vi "Interfaz grafica - corriente(1).vi"() -> ()   [LabVIEW 2016]
uses:
  Optotune Lens Driver 4 Labview package/Optotune Lens Driver 4 Labview package/Hello Optotune Lens (30.06.2015)/Calibration.ctl
  <vilib>/DAQmx/read.llb/DAQmx Read (Analog 1D Wfm NChan NSamp).vi
  <vilib>/Analysis/2dsp.llb/Decimate (single shot, DBL).vi
  <vilib>/Utility/file.llb/Read Delimited Spreadsheet (string).vi
  <vilib>/DAQmx/miscellaneous.llb/DAQmx Fill In Error Info.vi
  <vilib>/Waveform/WDTOps.llb/WDT Index Channel DBL.vi
  <vilib>/Analysis/2dsp.llb/Decimate (continuous, DBL).vi
  <vilib>/Instr/_visa.llb/VISA Configure Serial Port (Instr).vi
  <vilib>/Utility/file.llb/Write Delimited Spreadsheet (string).vi
  <vilib>/Waveform/WDTOps.llb/WDT Get Waveform Time Array DBL.vi
  <vilib>/Analysis/NI_AALPro.lvlib
panel:
  in  "Restablecer Iniciales":bool
  in  "Incremento":dbl=0.1 format="%#_13g"
  out "Potencia derecho":dbl
  out "error out 4":errorcluster
  out "error out 3":errorcluster
  out "error out 2":errorcluster
  in  "Tab Control 3":enum32{"WL", "Video"}(tab)
  out "Waveform length":dbl[][](graph)
  in  "Minimo escala Y":dbl format="%#_13g"
  in  "Maximo escala Y":dbl format="%#_13g"
  in  "Escala autom. Y":u8=1
  in  "Escala autom. X":u8=1
  in  "Maximo escala X":dbl
  in  "Minimo escala X":dbl
  out "Image Out":T1(plugin-control)
  in  "Frame Rate":u32=30
  in  "Modo de video":u16(ring)=21 items=["160x90 I420 30 fps", "160x90 MJPG 30 fps", "160x90 RGB24 30 fps", "160x120 I420 30 fps", "160x120 MJPG 30 fps", "160x120 RGB24 30 fps", "176x144 I420 30 fps", "176x144 MJPG 30 fps", "176x144 RGB24 30 fps", "320x180 I420 30 fps", "320x180 MJPG 30 fps", "320x180 RGB24 30 fps", "320x240  I420 30 fps", "320x240 MJPG 30 fps", "320x240 RGB24 30 fps", "352x288 I420 30 fps", "352x288 MJPG 30 fps", "352x288 RGB24 30 fps", "432x240 I420 30 fps", "432x240 MJPG 30 fps", "432x240 RGB24 30 fps", "640x360 I420 30 fps", "640x360 MJPG 30 fps", "640x360 RGB24 30 fps", "640x480 I420 30 fps", "640x480 MJPG 30 fps", "640x480 RGB24 30 fps", "800x448 I420 30 fps", "800x448 MJPG 30 fps", "800x448 RGB24 30 fps", "800x600 I420 30 fps", "800x600 MJPG 30 fps", "800x600 RGB24 30 fps", "864x480 I420 30 fps", "864x480 MJPG 30 fps", "864x480 RGB24 30 fps", "960x720 I420 30 fps", "960x720 MJPG 30 fps", "960x720 RGB24 30 fps", "1024x576 I420 30 fps", "1024x576 MJPG 30 fps", "1024x576 RGB24 30 fps", "1280x720 I420 30 fps", "1280x720 MJPG 30 fps", "1280x720 RGB24 30 fps", "1600x896 I420 30 fps", "1600x896 MJPG 30 fps", "1600x896 RGB24 30 fps", "1920x1080 I420 5 fps", "1920x1080 MJPG 30 fps", "1920x1080 RGB24 5 fps", "2304x1296 I420 2 fps", "2304x1296 RGB24 2 fps", "2304x1536 I420 2 fps", "2304x1536 RGB24 2 fps"]
  in  "Carpeta archivo":string="C:\\Users\\TGM1603\\Documents\\LabVIEW Data\\Experimentos electrodos\\VideosExperimentos"
  in  "Calidad":u32=1000
  out "VISA resource name out":string
  in  "Tab Control 2":T2(tab)
  in  "DAQmx Physical Channel":tag
  in  "Frecuencia muestreo":i32=20000
  in  "Rango voltaje":i16(ring)=5 items=["0.1"=0, "1"=1, "5"=5, "10"=10]
  in  "tamaño buffer":i32=1000
  in  "factor decimacion":i32=20
  in  "Ganancia":u16(ring) items=["0.2"=51455, "1"=33023, "10"=49407, "20"=41215, "30"=57599, "40"=37119, "60"=53503, "80"=45311, "120"=61695, "157"=35071, ""=0]
  in  "Potencia inicial lente derecho":dbl(slide) scale=-3.0..3.0
  in  "Potencia inicial lente izquierdo":dbl(slide) scale=-3.0..3.0
  in  "VISA resource name":string="COM11"
  in  "VISA resource name 2":string="COM10"
  out "DPT INICIALES D":dbl
  out "DPT INICIALES I":dbl
  out "Potencia izquierdo":dbl
  in  "error in (no error) 5":errorcluster
  in  "error in (no error) 4":errorcluster
  in  "error in (no error) 3":errorcluster
  in  "error in (no error) 2":errorcluster
  in  "Calibration 4":T3={"Max Current A"=293.0, "Max Current B"=293.0, "UCL A"=300.0, "UCL B"=300.0, "LCL A"=0.0, "LCL B"=0.0} {"Max Current A" format="%#_g mA"; "Max Current B" format="%#_g mA"; "UCL A" format="%#_g mA"; "LCL A" format="%#_g mA"; "UCL B" format="%#_g mA"; "LCL B" format="%#_g mA"}
  out "ID 2":u16
  out "VISA resource name out 2":string
  out "Calibration 3":T3 {"Max Current A" format="%#_g mA"; "Max Current B" format="%#_g mA"; "UCL A" format="%#_g mA"; "LCL A" format="%#_g mA"; "UCL B" format="%#_g mA"; "LCL B" format="%#_g mA"}
  out "OK 2":bool
  out "Data 2":string
  out "Command to Port 2":string
  in  "Cola tipo 2":dbl[](array[numeric])
  out "Distancia":u32
  in  "Tamaño ventana WL":i32=60
  in  "Limite inferior WL":dbl=25.0 format="%#_13g"
  in  "Limite superior WL":dbl=50.0
  out "number":u32
  in  "Calibration":T3={"Max Current A"=293.0, "Max Current B"=293.0, "UCL A"=300.0, "UCL B"=300.0, "LCL A"=0.0, "LCL B"=0.0} {"Max Current A" format="%#_g mA"; "Max Current B" format="%#_g mA"; "UCL A" format="%#_g mA"; "LCL A" format="%#_g mA"; "UCL B" format="%#_g mA"; "LCL B" format="%#_g mA"}
  out "ID":u16
  out "Calibration 2":T3 {"Max Current A" format="%#_g mA"; "Max Current B" format="%#_g mA"; "UCL A" format="%#_g mA"; "LCL A" format="%#_g mA"; "UCL B" format="%#_g mA"; "LCL B" format="%#_g mA"}
  out "OK":bool
  out "Data":string
  out "Command to Port":string
  in  "DPT dif.":dbl
  out "error out":errorcluster
  in  "error in (no error)":errorcluster
  in  "WL":dbl
  in  "Cola tipo":dbl[](array[numeric])
  out "T button?":bool
  in  "Elegir menu Exp":bool
  in  "Elegir menu":bool
  out "path":path
  in  "Iniciar experimento":bool
  in  "Parar adquisicion":bool
  out "Enfermedad visual":string
  out "Edad":string
  out "Nombre":string
  out "Cedula":string
  in  "Carpeta":path=path "C:/Users/TGM1603/Documents/LabVIEW Data/Experimentos electrodos"
  in  "?":bool
  in  "Menu Principal":u16(ring) items=["Visualizacion general ", "Llevar a cabo un experimento", "Ajustar potencia inicial lentes"]
  in  "Menu experimentos":u16(ring) items=["Experimento 1", "Experimento 2", "Experimento 3", "Experimento 4", "", "", "", ""]
  in  "Tab Control":enum32{"Señal EMG", "Potencia y distancia"}(tab)
  out "Senal EMG":waveform(dbl)[](graph)
  in  "Escala automatica Y":u8
  in  "Escala automatica X":u8=1
  in  "X Scale.Range:Increment":dbl
  in  "X Scale.Range:Minimum":dbl
  in  "X Scale.Range:Maximum":dbl
  in  "Y Scale.Range:Minimum":dbl=-5.0
  in  "Y Scale.Range:Maximum":dbl=5.0
  in  "Escala Y min":dbl
  in  "Escala Y max":dbl
  in  "Auto scale Y":u8=1
  in  "Escala X max":dbl
  in  "Escala X min":dbl
  out "Potencia optica y distancia":dbl[][](graph)
  in  "Auto scale X":u8=1
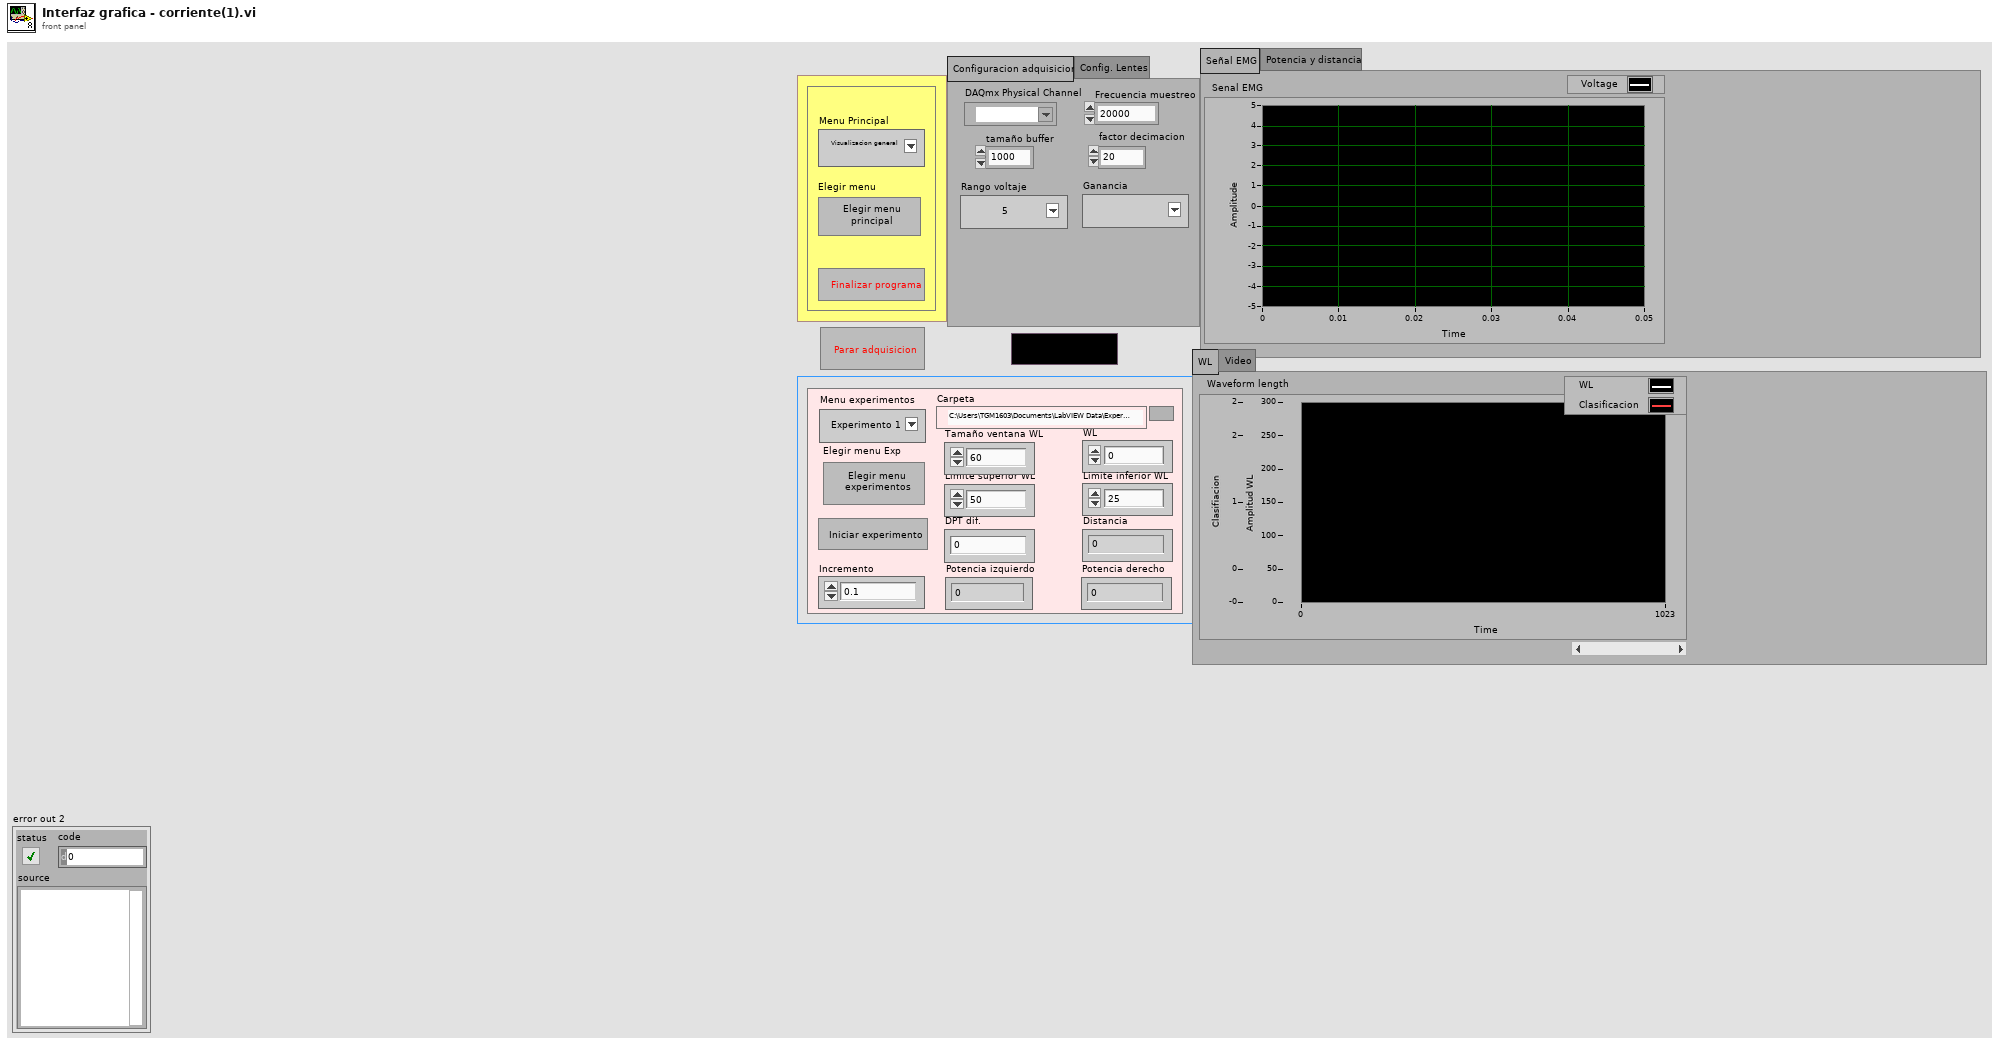
[diagram p1: front panel]
types:
  T1 = typedef "IMAQ Image.ctl" = refnum<image>
  T2 = enum32{"Configuracion adquisicion", "Config. Lentes"}
  T3 = typedef "Calibration.ctl" = cluster{"Max Current A":dbl, "Max Current B":dbl, "UCL A":dbl, "UCL B":dbl, "LCL A":dbl, "LCL B":dbl}
  T4 = enum16{"Left Button", "Center Button", "Right Button", "Window Close"}
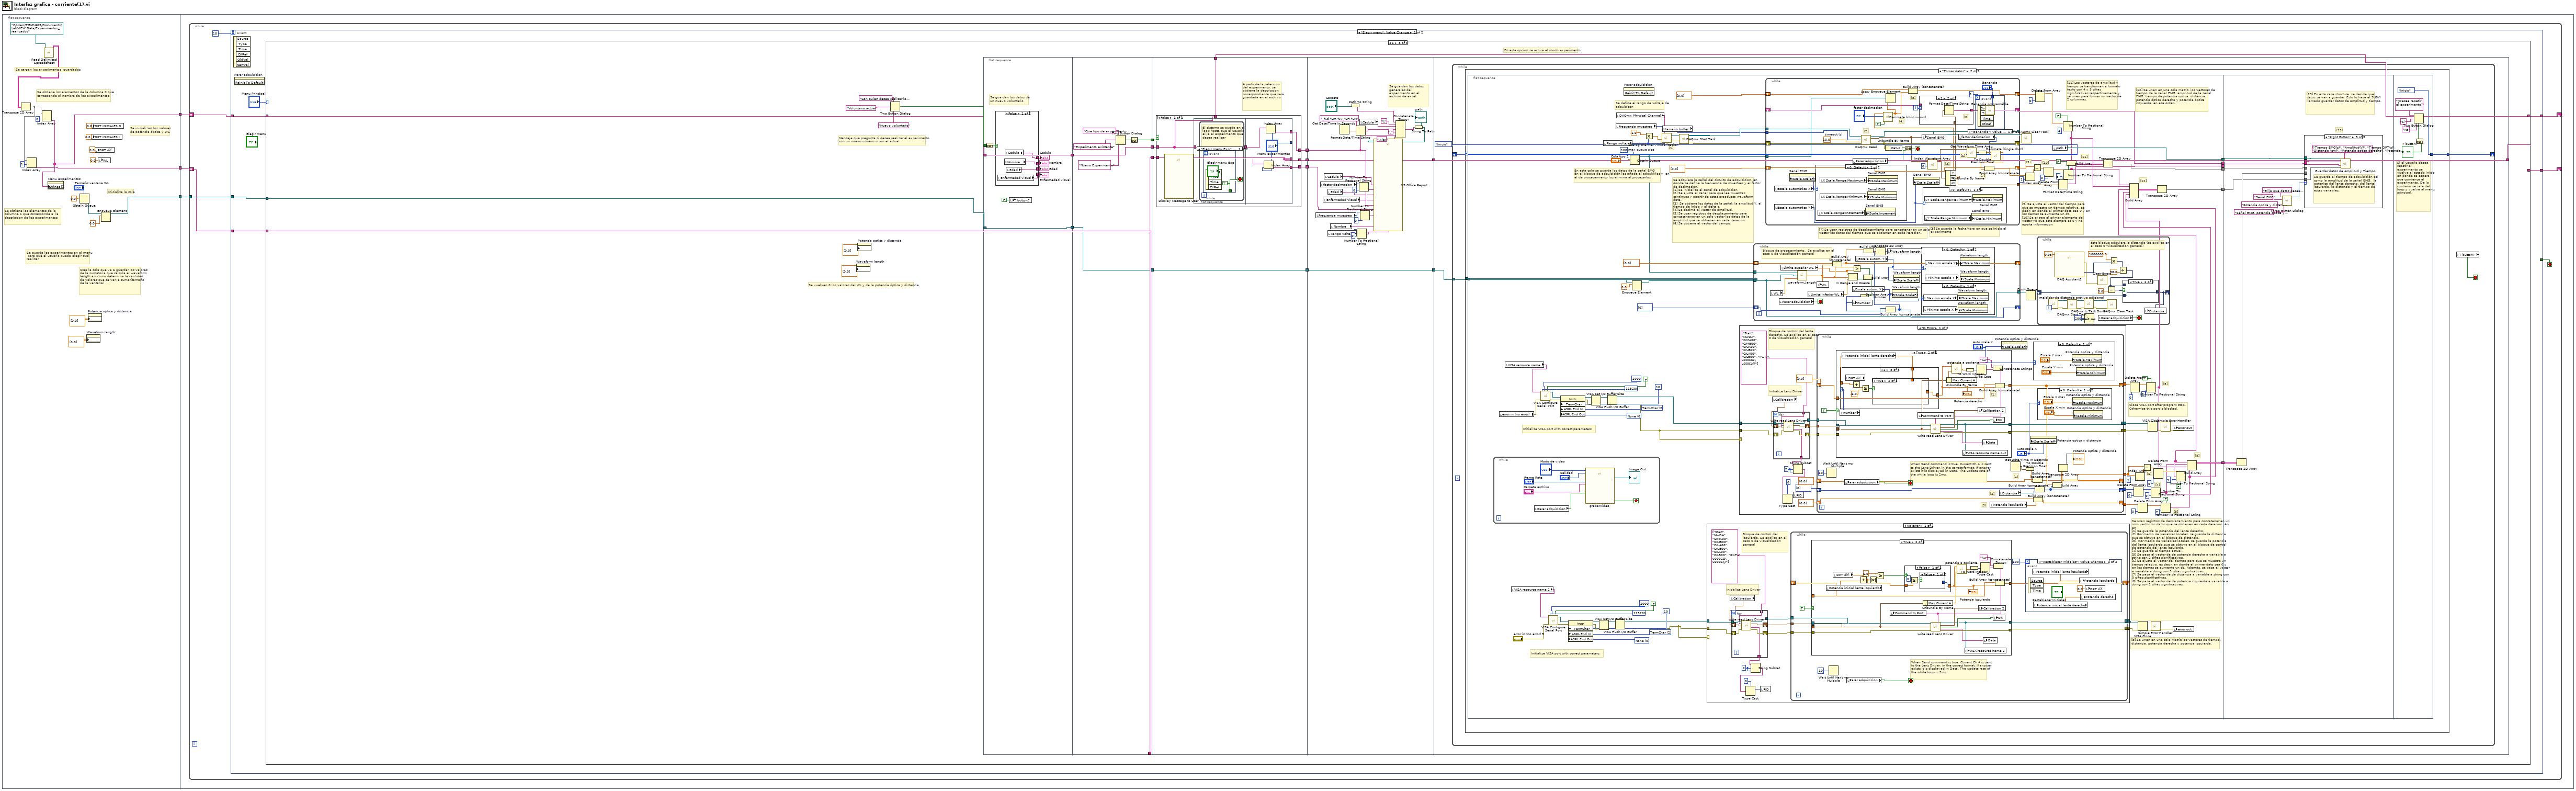
[diagram p0: block diagram]
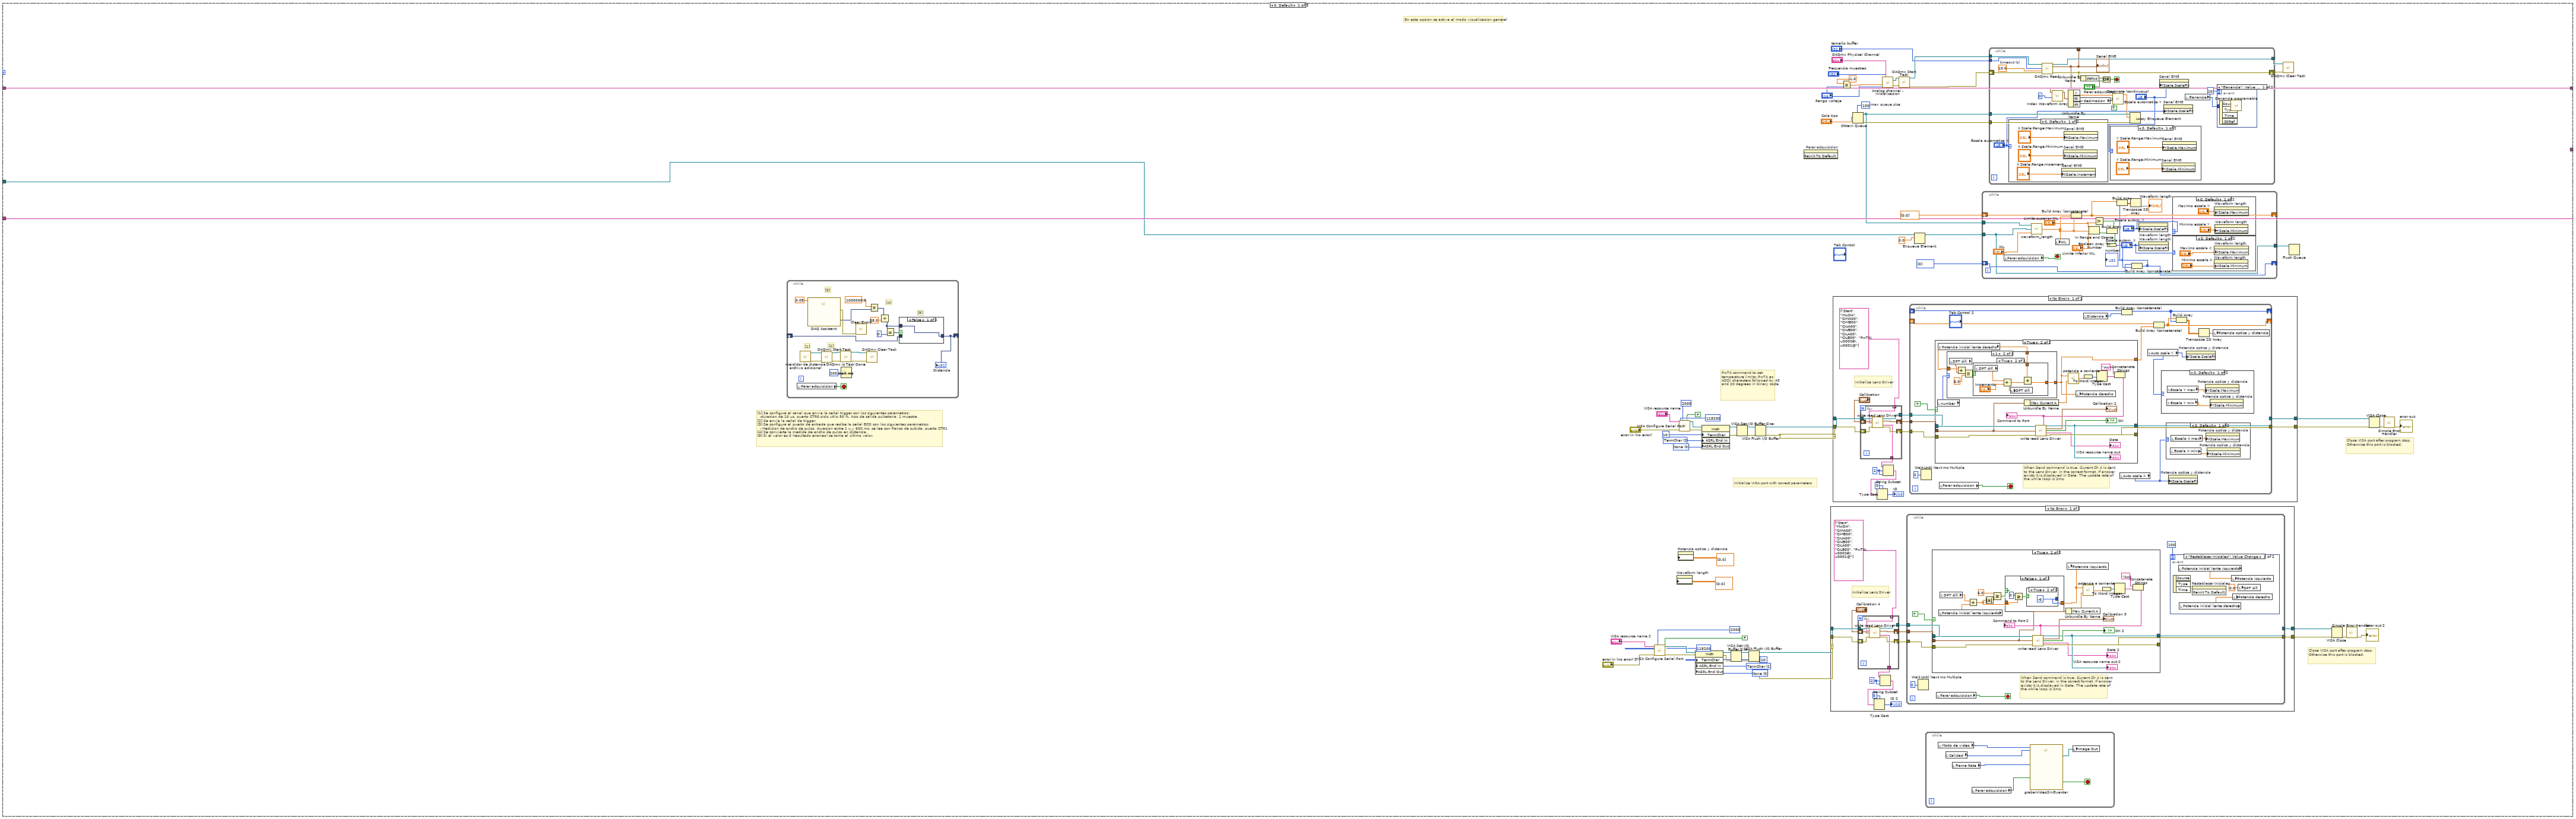
[diagram p2: hidden frame]
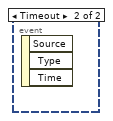
[diagram p3: hidden frame]
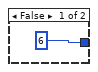
[diagram p5: hidden frame]
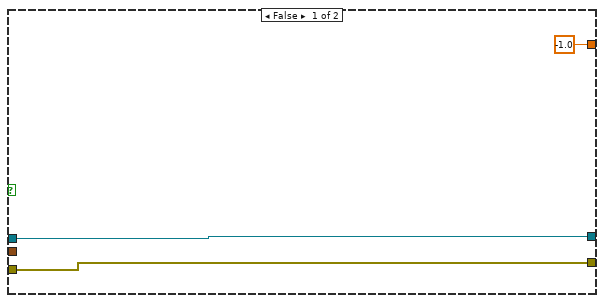
[diagram p11: hidden frame]
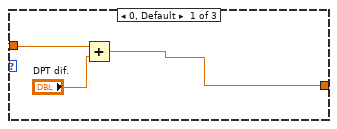
[diagram p12: hidden frame]
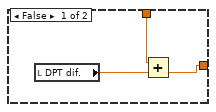
[diagram p13: hidden frame]
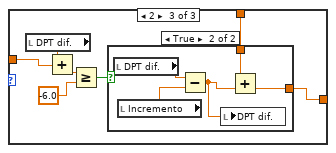
[diagram p14: hidden frame]
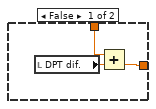
[diagram p15: hidden frame]
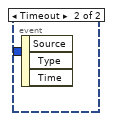
[diagram p19: hidden frame]
diagram:
  n1 = flat-sequence {
    tunnel: [w18] -> w3
    tunnel: [w15] -> w2
    tunnel: [w10] -> w1
    tunnel: w3 -> [w24]
    tunnel: w2 -> [w23]
    tunnel: w1 -> [w22]
    frame #0 {
      # "Se inicializan los valores\nde potencia óptica y WL"
      # "Inicializa la cola"
      # "Crea la cola que va a guardar los valores de la sumatoria que calcula el waveform length así como determina la cantidad de valores que se van a sumar(tamaño de la ventana)"
      # "Se obtiene los elementos de la columna 1 que corresponde a  la descripcion de los experimentos"
      # "Se obtiene los elementos de la columna 0 que corresponde al nombre de los experimentos"
      # "Se guarda los experimentos en el menu\n para que el usuario pueda elegir cual \nrealizar"
      # "Se cargan los experimentos  guardados"
      n2 = call-poly <vilib>:"Read Delimited Spreadsheet.vi"("file path (dialog if empty)"=path "C:/Users/TGM1603/Documents/LabVIEW Data/Experimentos_realizados") -> ("all rows"=w19:string[][])  [unwired: 9 in, 5 out]
      n3 = Transpose 2D Array(2D array=w19) -> (transposed array=w16:string[][])
      n4 = Index Array(array=w16, index (row)=1) -> (element=w15:string[])  [unwired: 1 in]
      n5 = Index Array(array=w16, index (row)=0) -> (element=w18:string[])  [unwired: 1 in]
      n6 = property on="Menu experimentos" class="Ring (strict)"("Strings []"=w18) -> ()  [unwired: 2 in, 2 out]
      n7 = Obtain Queue(max queue size (-1, unlimited)="Tamaño ventana WL", element data type=0.0) -> (queue out=w13:refnum<queue>)  [unwired: 3 in, 2 out]
      n8 = property on="Waveform length" class="WFChart (strict)"("History Data"=dbl[][] [[0.0]]) -> ()  [unwired: 2 in, 2 out]
      n9 = property on="Potencia optica y distancia" class="WFChart (strict)"("History Data"=dbl[][] [[0.0]]) -> ()  [unwired: 2 in, 2 out]
      n10 = local write "DPT INICIALES D"(0.0 ("DPT INIT.1")) -> ()
      n11 = local write "DPT INICIALES I"(0.0 ("DPT INIT.2")) -> ()
      n12 = local write "DPT dif."(0.0 ("WL")) -> ()
      n13 = local write "WL"(0.0 ("WL")) -> ()
      n14 = Enqueue Element(queue=w13, element=0.0) -> (queue out=w10:refnum<queue>)  [unwired: 2 in, 2 out]
    }
    frame #1 {
      n15 = while {
        shift-right: [w30] -> _
        shift-left: w24 -> [w31]
        shift-right: [w28] -> _
        shift-left: w23 -> [w29]
        tunnel: w22 -> [w27]
        stop <- w26 stop-if-true
        n16 = event shown="[0] \"Elegir menu\": Value Change" {
          selector: _ -> [_ _]
          dyn-events: _ -> [_ _]
          timeout: 10 -> [_ _]
          tunnel: w31 -> [w37 _]
          tunnel: [w36 _] -> w30
          tunnel: w29 -> [w35 _]
          tunnel: [w34 _] -> w28
          tunnel: w27 -> [w32 _]
          tunnel: [_ "?"] -> w26
          event "Elegir menu": Value Change {
            n17 = event-data() -> ()  [unwired: 1 in, 6 out]
            n18 = invoke on="Parar adquisicion" class="Bool (strict)" method="Reinit To Default"() -> ()  [unwired: 3 in, 3 out]
            n19 = case shown="1" "Menu Principal" {
              tunnel: w37 -> [w103 w388 w508]
              tunnel: [w103 w388 w507] -> w36
              tunnel: w35 -> [w102 w387 w505]
              tunnel: [w102 w387 w504] -> w34
              tunnel: w32 -> [w85 _ w495]
              frame 0, Default {
                w53 = u16 0 items=["None", "Last Bit", "TermChar", "Break"] ("Serial Settings:End Mode for Writes")
                w52 = u16 2 items=["None", "Last Bit", "TermChar"] ("Serial Settings:End Mode for Reads")
                w75 = u16 0 items=["None", "Last Bit", "TermChar", "Break"] ("Serial Settings:End Mode for Writes")
                w76 = u16 2 items=["None", "Last Bit", "TermChar"] ("Serial Settings:End Mode for Reads")
                w89 = 100  # max queue size
                # "En esta opcion se activa el modo visualizacion general"
                # "Close VISA port after program stop. Otherwise this port is blocked."
                # "[1] Se configura el canal que envía la señal trigger con los siguientes parametros:\n  -duracion de 10 us, puerto CTR0,ciclo utilo 50 %, tipo de salida pulsatoria, 1 muestra \n[2] Se envía la señal de trigger.\n[3] Se configura el puerto de entrada que recibe la señal ECO con los siguientes parámetros:\n  - Medicion de ancho de pulso, duracion entre 1 u y 600 ms, se lee con flanco de subida, puerto CTR1\n[4] Se convierte la medida de ancho de pulso en distancia.\n[5] Si el valor es 0 (resultado erroneo) se toma el último valor."
                # "PwTA command to set temperature limits: PwTA as ASCII characters followed by 45 and 20 degrees in binary code."
                # "Close VISA port after program stop. Otherwise this port is blocked."
                # "Initialize VISA port with correct parameters"
                n20 = while {
                  shift-right: [w177] -> _
                  shift-left: _ -> [w176]
                  stop <- w181 stop-if-true
                  # "[5]"
                  # "[4]"
                  # "[3]"
                  # "[2]"
                  # "[1]"
                  n21 = local read "Parar adquisicion"() -> (w181:bool)
                  n22 = call "meididor de distancia archivo adicional.vi"() -> ("error out"=w184:errorcluster, "task out"=w185:refnum<k21>)  [unwired: 10 in]
                  n23 = call "DAQ Assistant"("timeout (s)"=0.05) -> ("data"=w194:dynamicdata, "error out"=w182:errorcluster)  [unwired: 16 in, 1 out]
                  n24 = call <vilib>:"DAQmx Start Task.vi"("task/channels in"=w185, "error in"=w184) -> ("task out"=w188:refnum<k21>, "error out"=w189:errorcluster)  [unwired: 12 in]
                  n25 = call <vilib>:"DAQmx Is Task Done.vi"("task/channels in"=w188, "error in"=w189) -> ("task out"=w186:refnum<k21>, "error out"=w187:errorcluster)  [unwired: 11 in, 1 out]
                  n26 = Wait (ms)(milliseconds to wait=u32 200) -> ()  [unwired: 1 out]
                  n27 = call <vilib>:"Clear Errors.vi"("error in (no error)"=w182) -> ()  [unwired: 5 in, 2 out]
                  n28 = call <vilib>:"DAQmx Clear Task.vi"("task in"=w186, "error in"=w187) -> ()  [unwired: 13 in, 1 out]
                  n29 = Multiply(x=1000000.0, y=w194) -> (x*y=w192:dynamicdata)
                  n30 = Divide(x=w192, y=58.0) -> (x/y=w178:dynamicdata)
                  n31 = Equal?(x=w178, y=u16 0) -> (x = y?=w180:dynamicdata)
                  n32 = case shown="False" w180 {
                    tunnel: [w195 w196] -> w177
                    tunnel: w178 -> [w195 _]
                    tunnel: w176 -> [_ w196]
                    frame False {
                    }
                    frame True {
                    }
                  }
                  "Distancia" <- w177
                }
                n33 = call-poly "VISA Configure Serial Port"("VISA resource name"="VISA resource name 2", "timeout (10sec)"=u32 2000, "Enable Termination\nChar (T)"=FALSE ("Enable Termination\nChar (T)"), "baud rate (9600)"=u32 115200, "error in (no error)"="error in (no error) 2") -> ("VISA resource name out"=w48:refnum<visa-resource-name>, "error out"=w50:errorcluster)  [unwired: 9 in]
                n34 = property on="Waveform length" class="WFChart (strict)"("History Data"=dbl[][] [[0.0]]) -> ()  [unwired: 2 in, 2 out]
                n35 = property on="Potencia optica y distancia" class="WFChart (strict)"("History Data"=dbl[][] [[0.0]]) -> ()  [unwired: 2 in, 2 out]
                n36 = call-poly "VISA Configure Serial Port"("VISA resource name"="VISA resource name", "timeout (10sec)"=u32 2000, "Enable Termination\nChar (T)"=FALSE ("Enable Termination\nChar (T)"), "baud rate (9600)"=u32 115200, "error in (no error)"="error in (no error)") -> ("VISA resource name out"=w80:refnum<visa-resource-name>, "error out"=w78:errorcluster)  [unwired: 9 in]
                n37 = property class="Instr"(reference=w48, error in=w50, "TermChar"=u8 10 ("Message Based Settings:Termination Character"), "ASRL End In"=w52, "ASRL End Out"=w53) -> (reference out=w49:refnum<visa-resource-name>, error out=w51:errorcluster)
                n38 = property class="Instr"(reference=w80, error in=w78, "TermChar"=u8 10 ("Message Based Settings:Termination Character"), "ASRL End In"=w76, "ASRL End Out"=w75) -> (reference out=w79:refnum<visa-resource-name>, error out=w77:errorcluster)
                n39 = VISA Set I/O Buffer Size(VISA resource name=w49, error in (no error)=w51) -> (VISA resource name out=w56:refnum<visa-resource-name>, error out=w57:errorcluster)  [unwired: 2 in]
                n40 = VISA Set I/O Buffer Size(VISA resource name=w79, error in (no error)=w77) -> (VISA resource name out=w72:refnum<visa-resource-name>, error out=w71:errorcluster)  [unwired: 2 in]
                n41 = VISA Flush I/O Buffer(VISA resource name=w56, error in (no error)=w57) -> (VISA resource name out=w42:refnum<visa-resource-name>, error out=w43:errorcluster)  [unwired: 1 in]
                n42 = VISA Flush I/O Buffer(VISA resource name=w72, error in (no error)=w71) -> (VISA resource name out=w70:refnum<visa-resource-name>, error out=w65:errorcluster)  [unwired: 1 in]
                n43 = invoke on="Parar adquisicion" class="Bool (strict)" method="Reinit To Default"() -> ()  [unwired: 3 in, 3 out]
                n44 = case shown="No Error" w43 {
                  tunnel: w43 -> [w123 w174]
                  tunnel: w42 -> [w122 w175]
                  tunnel: [w121 w174] -> w38
                  tunnel: [w120 w175] -> w39
                  frame No Error {
                    w118 = 2 ("length (rest)")
                    # "Initialize Lens Driver"
                    n45 = for {
                      tunnel: w122 -> [w172]
                      tunnel: [w169] -> w112
                      tunnel: string[] ["Start", "MwDA", "CrMA00", "CrMB00", "CrUA00", "CrUB00", "CrLA00", "CrLB00", "PwTA\u0002Ð\u0001@"] -> [w167] mode=indexing
                      tunnel: [w166] -> w111
                      shift-right: [w170] -> w113
                      shift-left: "Calibration 4" -> [w171]
                      shift-right: [w168] -> w114
                      shift-left: w123 -> [w173]
                      n46 = call "write read Lens Driver.vi"("VISA resource name"=w172, "command"=w167, "Calibration"=w171, "error in (no error)"=w173) -> ("VISA resource name out"=w169:refnum<visa-resource-name>, "Calibration 2"=w170:T3, "Data"=w166:string, "error out"=w168:errorcluster)  [unwired: 4 in, 4 out]
                    }
                    n47 = String Subset(string=w111, offset (0)=w118, length (rest)=w118) -> (substring=w116:string)
                    n48 = Type Cast(type=u16 0 ("length (rest)"), x=w116) -> (*(type *) &x=→"ID 2":u16)
                    n49 = while {
                      tunnel: [w126] -> w121
                      tunnel: [w127] -> w120
                      tunnel: w114 -> [w132]
                      tunnel: w113 -> [w131]
                      tunnel: w112 -> [w130]
                      stop <- w125 stop-if-true
                      # "When Send command is true, Current Ch A is sent to the Lens Driver, in the correct format. If answer exists it is displayed in Data. The update rate of the while loop is 2ms."
                      n50 = Wait Until Next ms Multiple(millisecond multiple=u32 2) -> ()  [unwired: 1 out]
                      n51 = case shown="True" TRUE ("Send command") {
                        tunnel: [w137 w158] -> w126
                        tunnel: w132 -> [w137 w157]
                        tunnel: w131 -> [_ w139]
                        tunnel: w130 -> [w136 w156]
                        tunnel: [w136 w153] -> w127
                        frame False {
                        }
                        frame True {
                          n52 = local read "Potencia inicial lente izquierdo"() -> (w147:dbl)
                          n53 = local read "DPT dif."() -> (w148:dbl)
                          n54 = Add(x=w148, y=w147) -> (x+y=w143:dbl)
                          n55 = Absolute Value(x=w143) -> (abs(x)=w145:dbl)
                          n56 = Greater Or Equal?(x=6.0, y=w145) -> (x >= y?=w146:bool)
                          n57 = case shown="False" w146 {
                            tunnel: w143 -> [w161 w165]
                            tunnel: [w159 w165] -> w141
                            frame False {
                              n58 = Greater Or Equal?(x=u16 0, y=w161) -> (x >= y?=w162:bool)
                              n59 = case shown="True" w162 {
                                tunnel: [i16 6 ("x") i16 -6 ("x")] -> w159
                                frame False {
                                }
                                frame True {
                                }
                              }
                            }
                            frame True {
                            }
                          }
                          n60 = Unbundle By Name(w139) -> ("Max Current A"=w140:dbl)
                          n61 = local write "Potencia izquierdo"(w141) -> ()
                          n62 = call "potencia a corriente.vi"("Max current A"=w140, "Potencia"=w141) -> ("Corriente"=w142:dbl)
                          n63 = To Word Integer(number=w142) -> (16bit integer=w151:i16)
                          n64 = Type Cast(x=w151) -> (*(type *) &x=w150:string)  [unwired: 1 in]
                          n65 = Concatenate Strings("Aw", w150) -> (w149:string)
                          "Command to Port 2" <- w149
                          n66 = call "write read Lens Driver.vi"("VISA resource name"=w156, "command"=w149, "Calibration"=w139, "error in (no error)"=w157) -> ("VISA resource name out"=w153:refnum<visa-resource-name>, "Calibration 2"=→"Calibration 3":T3, "OK"=→"OK 2":bool, "Data"=→"Data 2":string, "error out"=w158:errorcluster)  [unwired: 4 in, 3 out]
                          "VISA resource name out 2" <- w153
                        }
                      }
                      n67 = local read "Parar adquisicion"() -> (w125:bool)
                      n68 = event shown="[0] \"Restablecer Iniciales\": Value Change" {
                        selector: _ -> [_ _]
                        dyn-events: _ -> [_ _]
                        timeout: 100 -> [_ _]
                        event "Restablecer Iniciales": Value Change {
                          n69 = event-data() -> ()  [unwired: 1 in, 3 out]
                          n70 = local read "Potencia inicial lente izquierdo"() -> (w133:dbl)
                          n71 = local read "Potencia inicial lente derecho"() -> (w134:dbl)
                          n72 = invoke on="Restablecer Iniciales" class="Bool" method="Reinit To Default"() -> ()  [unwired: 3 in, 3 out]
                          n73 = local write "Potencia izquierdo"(w133) -> ()
                          n74 = local write "Potencia derecho"(w134) -> ()
                          n75 = local write "DPT dif."(0.0 ("DPT dif.")) -> ()
                        }
                        event Timeout {
                          n76 = event-data() -> ()  [unwired: 1 in, 3 out]
                        }
                      }
                    }
                  }
                  frame Error {
                  }
                }
                n77 = case shown="No Error" w65 {
                  tunnel: w65 -> [w210 w294]
                  tunnel: w70 -> [w209 w295]
                  tunnel: [w208 w294] -> w68
                  tunnel: [w207 w295] -> w66
                  frame No Error {
                    w205 = 2 ("length (rest)")
                    # "Initialize Lens Driver"
                    n78 = for {
                      tunnel: w209 -> [w292]
                      tunnel: [w289] -> w199
                      tunnel: string[] ["Start", "MwDA", "CrMA00", "CrMB00", "CrUA00", "CrUB00", "CrLA00", "CrLB00", "PwTA\u0002Ð\u0001@"] -> [w287] mode=indexing
                      tunnel: [w286] -> w198
                      shift-right: [w290] -> w200
                      shift-left: "Calibration" -> [w291]
                      shift-right: [w288] -> w201
                      shift-left: w210 -> [w293]
                      n79 = call "write read Lens Driver.vi"("VISA resource name"=w292, "command"=w287, "Calibration"=w291, "error in (no error)"=w293) -> ("VISA resource name out"=w289:refnum<visa-resource-name>, "Calibration 2"=w290:T3, "Data"=w286:string, "error out"=w288:errorcluster)  [unwired: 4 in, 4 out]
                    }
                    n80 = String Subset(string=w198, offset (0)=w205, length (rest)=w205) -> (substring=w203:string)
                    n81 = Type Cast(type=u16 0 ("length (rest)"), x=w203) -> (*(type *) &x=→"ID":u16)
                    n82 = while {
                      tunnel: [w222] -> w208
                      tunnel: [w223] -> w207
                      tunnel: w201 -> [w228]
                      tunnel: w200 -> [w227]
                      tunnel: w199 -> [w226]
                      shift-right: [w213] -> _
                      shift-left: _ -> [w217]
                      shift-right: [w214] -> _
                      shift-left: _ -> [w216]
                      stop <- w221 stop-if-true
                      # "When Send command is true, Current Ch A is sent to the Lens Driver, in the correct format. If answer exists it is displayed in Data. The update rate of the while loop is 2ms."
                      n83 = Wait Until Next ms Multiple(millisecond multiple=u32 2) -> ()  [unwired: 1 out]
                      n84 = case shown="True" TRUE ("Send command") {
                        tunnel: [w235 w252] -> w222
                        tunnel: w228 -> [w235 w251]
                        tunnel: w227 -> [_ w238]
                        tunnel: w226 -> [w234 w250]
                        tunnel: [w234 w247] -> w223
                        tunnel: [-1.0 ("DPT") w240] -> w215
                        frame False {
                        }
                        frame True {
                          n85 = local read "number"() -> (w242:u32)
                          n86 = local read "Potencia inicial lente derecho"() -> (w241:dbl)
                          n87 = case shown="1" w242 {
                            tunnel: [w254 w262 w277] -> w240
                            tunnel: w241 -> [w255 w257 w272]
                            tunnel: w241 -> [_ w256 w271]
                            frame 0, Default {
                              n88 = Add(x=w255, y="DPT dif.") -> (x+y=w254:dbl)
                            }
                            frame 1 {
                              n89 = local read "DPT dif."() -> (w258:dbl)
                              n90 = Add(x=w257, y=w258) -> (x+y=w259:dbl)
                              n91 = Less Or Equal?(x=w259, y=6.0) -> (x <= y?=w261:bool)
                              n92 = case shown="True" w261 {
                                tunnel: [w264 w267] -> w262
                                tunnel: w256 -> [w263 w266]
                                frame False {
                                n93 = local read "DPT dif."() -> (w265:dbl)
                                n94 = Add(x=w263, y=w265) -> (x+y=w264:dbl)
                                }
                                frame True {
                                n95 = local read "DPT dif."() -> (w268:dbl)
                                n96 = Add(x=w268, y="Incremento") -> (x+y=w269:dbl)
                                n97 = local write "DPT dif."(w269) -> ()
                                n98 = Add(x=w266, y=w269) -> (x+y=w267:dbl)
                                }
                              }
                            }
                            frame 2 {
                              n99 = local read "DPT dif."() -> (w276:dbl)
                              n100 = Add(x=w276, y=w272) -> (x+y=w273:dbl)
                              n101 = Greater Or Equal?(x=w273, y=-6.0) -> (x >= y?=w274:bool)
                              n102 = case shown="True" w274 {
                                tunnel: [w279 w283] -> w277
                                tunnel: w271 -> [w278 w282]
                                frame False {
                                n103 = local read "DPT dif."() -> (w280:dbl)
                                n104 = Add(x=w278, y=w280) -> (x+y=w279:dbl)
                                }
                                frame True {
                                n105 = local read "DPT dif."() -> (w285:dbl)
                                n106 = local read "Incremento"() -> (w281:dbl)
                                n107 = Subtract(x=w285, y=w281) -> (x-y=w284:dbl)
                                n108 = local write "DPT dif."(w284) -> ()
                                n109 = Add(x=w282, y=w284) -> (x+y=w283:dbl)
                                }
                              }
                            }
                          }
                          n110 = Unbundle By Name(w238) -> ("Max Current A"=w237:dbl)
                          n111 = call "potencia a corriente.vi"("Max current A"=w237, "Potencia"=w240) -> ("Corriente"=w239:dbl)
                          n112 = local write "Potencia derecho"(w240) -> ()
                          n113 = To Word Integer(number=w239) -> (16bit integer=w245:i16)
                          n114 = Type Cast(x=w245) -> (*(type *) &x=w244:string)  [unwired: 1 in]
                          n115 = Concatenate Strings("Aw", w244) -> (w243:string)
                          "Command to Port" <- w243
                          n116 = call "write read Lens Driver.vi"("VISA resource name"=w250, "command"=w243, "Calibration"=w238, "error in (no error)"=w251) -> ("VISA resource name out"=w247:refnum<visa-resource-name>, "Calibration 2"=→"Calibration 2":T3, "OK"=→"OK":bool, "Data"=→"Data":string, "error out"=w252:errorcluster)  [unwired: 4 in, 3 out]
                          "VISA resource name out" <- w247
                        }
                      }
                      n117 = local read "Parar adquisicion"() -> (w221:bool)
                      n118 = local read "Distancia"() -> (w218:u32)
                      n119 = local read "Auto scale X"() -> (w219:u8)
                      n120 = Build Array (concatenate)(w217, w218) -> (w213:u32[])
                      n121 = local read "Auto scale Y"() -> (w220:u8)
                      n122 = Build Array (concatenate)(w216, w215) -> (w214:dbl[])
                      n123 = case shown="0, Default" w220 {
                        frame 0, Default {
                          n124 = local read "Escala Y min"() -> (w231:dbl)
                          n125 = local read "Escala Y max"() -> (w232:dbl)
                          n126 = property on="Potencia optica y distancia" class="WFChart (strict)"("YScale.Maximum"=w232) -> ()  [unwired: 2 in, 2 out]
                          n127 = property on="Potencia optica y distancia" class="WFChart (strict)"("YScale.Minimum"=w231) -> ()  [unwired: 2 in, 2 out]
                        }
                        frame 1 {
                        }
                      }
                      n128 = case shown="0, Default" w219 {
                        frame 0, Default {
                          n129 = local read "Escala X min"() -> (w229:dbl)
                          n130 = local read "Escala X max"() -> (w230:dbl)
                          n131 = property on="Potencia optica y distancia" class="WFChart (strict)"("XScale.Maximum"=w230) -> ()  [unwired: 2 in, 2 out]
                          n132 = property on="Potencia optica y distancia" class="WFChart (strict)"("XScale.Minimum"=w229) -> ()  [unwired: 2 in, 2 out]
                        }
                        frame 1 {
                        }
                      }
                      n133 = property on="Potencia optica y distancia" class="WFChart (strict)"("XScale.ScaleFit"=w219) -> ()  [unwired: 2 in, 2 out]
                      n134 = Build Array(w214, w213) -> (w212:dbl[][])
                      n135 = property on="Potencia optica y distancia" class="WFChart (strict)"("YScale.ScaleFit"=w220) -> ()  [unwired: 2 in, 2 out]
                      n136 = Transpose 2D Array(2D array=w212) -> (transposed array=w211:dbl[][])
                      n137 = local write "Potencia optica y distancia"(w211) -> ()
                    }
                  }
                  frame Error {
                  }
                }
                n138 = Multiply(x=-1.0 ("y"), y="Rango voltaje") -> (x*y=w92:dbl)
                n139 = Obtain Queue(max queue size (-1, unlimited)=w89, element data type="Cola tipo") -> (queue out=w86:refnum<queue>, error out=w87:errorcluster)  [unwired: 3 in, 1 out]
                n140 = call "Analog channel - inicializacion.vi"("maximum value"="Rango voltaje", "minimum value"=w92, "rate"="Frecuencia muestreo", "DAQmx Physical Channel"="DAQmx Physical Channel") -> ("error out"=w95:errorcluster, "task out"=w96:refnum<k21>)
                n141 = call <vilib>:"DAQmx Start Task.vi"("task/channels in"=w96, "error in"=w95) -> ("task out"=w101:refnum<k21>, "error out"=w100:errorcluster)  [unwired: 12 in]
                n142 = Enqueue Element(queue=w85, element=0.0) -> (queue out=w62:refnum<queue>)  [unwired: 2 in, 2 out]
                n143 = while {
                  stop <- w109 stop-if-true
                  n144 = local read "Modo de video"() -> (w105:u16)
                  n145 = local read "Calidad"() -> (w106:u32)
                  n146 = local read "Frame Rate"() -> (w107:u32)
                  n147 = local read "Parar adquisicion"() -> (w108:bool)
                  n148 = call "grabarVideoSinGuardar.vi"("VideoMode"=w105, "Quality"=w106, "Stop (F)"=w108, "Frame Rate"=w107) -> ("Image Out"=w104:T1, "Stopped"=w109:bool)  [unwired: 21 in, 1 out]
                  n149 = local write "Image Out"(w104) -> ()
                }
                n150 = while {
                  tunnel: w62 -> [w297]
                  tunnel: w86 -> [w314]
                  shift-right: [w300] -> _
                  shift-left: dbl[] [0.0] -> [w311]
                  shift-right: [w299] -> _
                  shift-left: u32[] [0] -> [w301]
                  tunnel: [w297] -> w60
                  stop <- w312 stop-if-true
                  n151 = local read "Parar adquisicion"() -> (w312:bool)
                  n152 = call "waveform_length.vi"("WL"="WL", "Cola WL"=w297, "Datos entrada"=w314) -> ("WL 2"=w309:dbl)
                  n153 = local write "WL"(w309) -> ()
                  n154 = Build Array (concatenate)(w311, w309) -> (w300:dbl[])
                  n155 = In Range and Coerce(upper limit="Limite superior WL", x=w309, lower limit="Limite inferior WL") -> (In Range?=w307:bool)  [unwired: 1 out]
                  n156 = Greater?(x=w309, y="Limite superior WL") -> (0:w308:bool)
                  n157 = Build Array(w308, w307) -> (w306:bool[])
                  n158 = Boolean Array To Number(Boolean array=w306) -> (number=w302:u32)
                  "number" <- w302
                  n159 = Build Array (concatenate)(w301, w302) -> (w299:u32[])
                  n160 = Build Array(w300, w299) -> (w298:dbl[][])
                  n161 = Transpose 2D Array(2D array=w298) -> (transposed array=→"Waveform length":dbl[][])
                  n162 = property on="Waveform length" class="WFChart (strict)"("YScale.ScaleFit"="Escala autom. Y") -> ()  [unwired: 2 in, 2 out]
                  n163 = property on="Waveform length" class="WFChart (strict)"("XScale.ScaleFit"="Escala autom. X") -> ()  [unwired: 2 in, 2 out]
                  n164 = case shown="0, Default" "Escala autom. Y" {
                    frame 0, Default {
                      n165 = property on="Waveform length" class="WFChart (strict)"("YScale.Maximum"="Maximo escala Y") -> ()  [unwired: 2 in, 2 out]
                      n166 = property on="Waveform length" class="WFChart (strict)"("YScale.Minimum"="Minimo escala Y") -> ()  [unwired: 2 in, 2 out]
                    }
                    frame 1 {
                    }
                  }
                  n167 = case shown="0, Default" "Escala autom. X" {
                    frame 0, Default {
                      n168 = property on="Waveform length" class="WFChart (strict)"("XScale.Maximum"="Maximo escala X") -> ()  [unwired: 2 in, 2 out]
                      n169 = property on="Waveform length" class="WFChart (strict)"("XScale.Minimum"="Minimo escala X") -> ()  [unwired: 2 in, 2 out]
                    }
                    frame 1 {
                    }
                  }
                }
                n170 = while {
                  tunnel: w101 -> [w340]
                  tunnel: "tamaño buffer" -> [w337]
                  tunnel: [w338] -> w97
                  shift-right: [w335] -> w98
                  shift-left: w100 -> [w339]
                  tunnel: [w329] -> _
                  tunnel: w86 -> [w325]
                  tunnel: w87 -> [w324]
                  stop <- w334 stop-if-true
                  w333 = 10.0  # timeout (s)
                  n171 = case shown="0, Default" "Escala automatica X" {
                    frame 0, Default {
                      n172 = property on="Senal EMG" class="WFGraph (strict)"("XScale.Increment"="X Scale.Range:Increment") -> ()  [unwired: 2 in, 2 out]
                      n173 = property on="Senal EMG" class="WFGraph (strict)"("XScale.Minimum"="X Scale.Range:Minimum") -> ()  [unwired: 2 in, 2 out]
                      n174 = property on="Senal EMG" class="WFGraph (strict)"("XScale.Maximum"="X Scale.Range:Maximum") -> ()  [unwired: 2 in, 2 out]
                    }
                    frame 1 {
                    }
                  }
                  n175 = call-poly <vilib>:"DAQmx Read.vi"("task/channels in"=w340, "number of samples per channel"=w337, "timeout"=w333, "error in"=w339) -> ("task out"=w338:refnum<k21>, "data"=w329:waveform(dbl)[], "error out"=w335:errorcluster)  [unwired: 9 in]
                  "Senal EMG" <- w329
                  n176 = call-poly <vilib>:"Index Waveform Array.vi"("index"=0, "waveform array"=w329) -> ("waveform"=w330:waveform(dbl))  [unwired: 8 in, 1 out]
                  n177 = Unbundle By Name(w330) -> ("Y"=w327:dbl[])  [unwired: 2 out]
                  n178 = local read "factor decimacion"() -> (w326:i32)
                  n179 = Unbundle By Name(w335) -> ("status"=w336:bool)
                  n180 = Or(x=w336, y="Parar adquisicion") -> (x .or. y?=w334:bool)
                  n181 = case shown="0, Default" "Escala automatica Y" {
                    frame 0, Default {
                      n182 = property on="Senal EMG" class="WFGraph (strict)"("YScale.Minimum"="Y Scale.Range:Minimum") -> ()  [unwired: 2 in, 2 out]
                      n183 = property on="Senal EMG" class="WFGraph (strict)"("YScale.Maximum"="Y Scale.Range:Maximum") -> ()  [unwired: 2 in, 2 out]
                    }
                    frame 1 {
                    }
                  }
                  n184 = call-poly <vilib>:"Decimate (continuous).vi"("averaging"=TRUE, "decimating factor"=w326, "X"=w327) -> ("Decimated Array"=w323:dbl[])  [unwired: 7 in, 1 out]
                  n185 = Lossy Enqueue Element(queue=w325, element=w323, error in (no error)=w324) -> ()  [unwired: 4 out]
                  n186 = property on="Senal EMG" class="WFGraph (strict)"("YScale.ScaleFit"="Escala automatica Y") -> ()  [unwired: 2 in, 2 out]
                  n187 = property on="Senal EMG" class="WFGraph (strict)"("XScale.ScaleFit"="Escala automatica X") -> ()  [unwired: 2 in, 2 out]
                  n188 = local read "Ganancia"() -> (w320:u16)
                  n189 = event shown="[0] \"Ganancia\": Value Change" {
                    selector: _ -> [_ _]
                    dyn-events: _ -> [_ _]
                    timeout: 10 -> [_ _]
                    tunnel: w320 -> [w341 _]
                    event "Ganancia": Value Change {
                      n190 = event-data() -> ()  [unwired: 1 in, 4 out]
                      n191 = call "Ganancia programable.vi"("MOSI data"=w341) -> ()
                    }
                    event Timeout {
                      n192 = event-data() -> ()  [unwired: 1 in, 3 out]
                    }
                  }
                }
                n193 = call <vilib>:"DAQmx Clear Task.vi"("task in"=w97, "error in"=w98) -> ()  [unwired: 13 in, 1 out]
                n194 = Flush Queue(queue=w60) -> ()  [unwired: 1 in, 3 out]
                n195 = VISA Close(VISA resource name=w39, error in (no error)=w38) -> (error out=w40:errorcluster)
                n196 = call <vilib>:"Simple Error Handler.vi"("error in (no error)"=w40) -> ("error out"=→"error out 2":errorcluster)  [unwired: 4 in, 4 out]
                n197 = VISA Close(VISA resource name=w66, error in (no error)=w68) -> (error out=w69:errorcluster)
                n198 = call <vilib>:"Simple Error Handler.vi"("error in (no error)"=w69) -> ("error out"=→"error out":errorcluster)  [unwired: 4 in, 4 out]
              }
              frame 2 {
                w367 = u16 0 items=["None", "Last Bit", "TermChar", "Break"] ("Serial Settings:End Mode for Writes")
                w366 = u16 2 items=["None", "Last Bit", "TermChar"] ("Serial Settings:End Mode for Reads")
                w380 = u16 0 items=["None", "Last Bit", "TermChar", "Break"] ("Serial Settings:End Mode for Writes")
                w379 = u16 2 items=["None", "Last Bit", "TermChar"] ("Serial Settings:End Mode for Reads")
                # "En esta opcion se configura la potencia inicial de los lentes"
                # "Close VISA port after program stop. Otherwise this port is blocked."
                # "Close VISA port after program stop. Otherwise this port is blocked."
                # "PwTA command to set temperature limits: PwTA as ASCII characters followed by 45 and 20 degrees in binary code."
                # "Initialize VISA port with correct parameters"
                # "PwTA command to set temperature limits: PwTA as ASCII characters followed by 45 and 20 degrees in binary code."
                # "Initialize VISA port with correct parameters"
                n199 = local read "VISA resource name"() -> (w357:string)
                n200 = call-poly "VISA Configure Serial Port"("VISA resource name"=w357, "timeout (10sec)"=u32 2000, "Enable Termination\nChar (T)"=FALSE ("Enable Termination\nChar (T)"), "baud rate (9600)"=u32 115200, "error in (no error)"="error in (no error) 3") -> ("VISA resource name out"=w362:refnum<visa-resource-name>, "error out"=w364:errorcluster)  [unwired: 9 in]
                n201 = property class="Instr"(reference=w362, error in=w364, "TermChar"=u8 10 ("Message Based Settings:Termination Character"), "ASRL End In"=w366, "ASRL End Out"=w367) -> (reference out=w363:refnum<visa-resource-name>, error out=w365:errorcluster)
                n202 = VISA Set I/O Buffer Size(VISA resource name=w363, error in (no error)=w365) -> (VISA resource name out=w369:refnum<visa-resource-name>, error out=w370:errorcluster)  [unwired: 2 in]
                n203 = VISA Flush I/O Buffer(VISA resource name=w369, error in (no error)=w370) -> (VISA resource name out=w356:refnum<visa-resource-name>, error out=w355:errorcluster)  [unwired: 1 in]
                n204 = case shown="No Error" w355 {
                  tunnel: w355 -> [w402 w436]
                  tunnel: w356 -> [w401 w437]
                  tunnel: [w400 w436] -> w351
                  tunnel: [w399 w437] -> w352
                  frame No Error {
                    w398 = 2 ("length (rest)")
                    # "Initialize Lens Driver"
                    n205 = local read "Calibration"() -> (w390:T3)
                    n206 = for {
                      tunnel: w401 -> [w434]
                      tunnel: [w431] -> w393
                      tunnel: string[] ["Start", "MwDA", "CrMA00", "CrMB00", "CrUA00", "CrUB00", "CrLA00", "CrLB00", "PwTA\u0002Ð\u0001@"] -> [w429] mode=indexing
                      tunnel: [w428] -> w392
                      shift-right: [w432] -> w394
                      shift-left: w390 -> [w433]
                      shift-right: [w430] -> w395
                      shift-left: w402 -> [w435]
                      n207 = call "write read Lens Driver.vi"("VISA resource name"=w434, "command"=w429, "Calibration"=w433, "error in (no error)"=w435) -> ("VISA resource name out"=w431:refnum<visa-resource-name>, "Calibration 2"=w432:T3, "Data"=w428:string, "error out"=w430:errorcluster)  [unwired: 4 in, 4 out]
                    }
                    n208 = String Subset(string=w392, offset (0)=w398, length (rest)=w398) -> (substring=w396:string)
                    n209 = Type Cast(type=u16 0 ("length (rest)"), x=w396) -> (*(type *) &x=w391:u16)
                    n210 = local write "ID"(w391) -> ()
                    n211 = while {
                      tunnel: [w404] -> w400
                      tunnel: [w405] -> w399
                      tunnel: w395 -> [w410]
                      tunnel: w394 -> [w409]
                      tunnel: w393 -> [w408]
                      stop <- w403 stop-if-true
                      # "When Send command is true, Current Ch A is sent to the Lens Driver, in the correct format. If answer exists it is displayed in Data. The update rate of the while loop is 2ms."
                      n212 = Wait Until Next ms Multiple(millisecond multiple=u32 2) -> ()  [unwired: 1 out]
                      n213 = case shown="True" TRUE ("Send command") {
                        tunnel: [w412 w427] -> w404
                        tunnel: w410 -> [w412 w426]
                        tunnel: w409 -> [_ w417]
                        tunnel: w408 -> [w411 w425]
                        tunnel: [w411 w418] -> w405
                        frame False {
                        }
                        frame True {
                          n214 = Unbundle By Name(w417) -> ("Max Current A"=w416:dbl)
                          n215 = call "potencia a corriente.vi"("Max current A"=w416, "Potencia"="Potencia inicial lente derecho") -> ("Corriente"=w414:dbl)
                          n216 = To Word Integer(number=w414) -> (16bit integer=w424:i16)
                          n217 = Type Cast(x=w424) -> (*(type *) &x=w423:string)  [unwired: 1 in]
                          n218 = Concatenate Strings("Aw", w423) -> (w420:string)
                          n219 = local write "Command to Port"(w420) -> ()
                          n220 = call "write read Lens Driver.vi"("VISA resource name"=w425, "command"=w420, "Calibration"=w417, "error in (no error)"=w426) -> ("VISA resource name out"=w418:refnum<visa-resource-name>, "Calibration 2"=w422:T3, "OK"=w421:bool, "Data"=w419:string, "error out"=w427:errorcluster)  [unwired: 4 in, 3 out]
                          n221 = local write "VISA resource name out"(w418) -> ()
                          n222 = local write "Calibration 2"(w422) -> ()
                          n223 = local write "Data"(w419) -> ()
                          n224 = local write "OK"(w421) -> ()
                          "DPT INICIALES D" <- "Potencia inicial lente derecho"
                        }
                      }
                      n225 = local read "Parar adquisicion"() -> (w403:bool)
                    }
                  }
                  frame Error {
                  }
                }
                n226 = VISA Close(VISA resource name=w352, error in (no error)=w351) -> (error out=w354:errorcluster)
                n227 = call <vilib>:"Simple Error Handler.vi"("error in (no error)"=w354) -> ("error out"=→"error out 3":errorcluster)  [unwired: 4 in, 4 out]
                n228 = local read "VISA resource name 2"() -> (w371:string)
                n229 = call-poly "VISA Configure Serial Port"("VISA resource name"=w371, "timeout (10sec)"=u32 2000, "Enable Termination\nChar (T)"=FALSE ("Enable Termination\nChar (T)"), "baud rate (9600)"=u32 115200, "error in (no error)"="error in (no error) 4") -> ("VISA resource name out"=w375:refnum<visa-resource-name>, "error out"=w377:errorcluster)  [unwired: 9 in]
                n230 = property class="Instr"(reference=w375, error in=w377, "TermChar"=u8 10 ("Message Based Settings:Termination Character"), "ASRL End In"=w379, "ASRL End Out"=w380) -> (reference out=w376:refnum<visa-resource-name>, error out=w378:errorcluster)
                n231 = VISA Set I/O Buffer Size(VISA resource name=w376, error in (no error)=w378) -> (VISA resource name out=w382:refnum<visa-resource-name>, error out=w383:errorcluster)  [unwired: 2 in]
                n232 = VISA Flush I/O Buffer(VISA resource name=w382, error in (no error)=w383) -> (VISA resource name out=w385:refnum<visa-resource-name>, error out=w384:errorcluster)  [unwired: 1 in]
                n233 = case shown="No Error" w384 {
                  tunnel: w384 -> [w451 w491]
                  tunnel: w385 -> [w450 w492]
                  tunnel: [w449 w491] -> w348
                  tunnel: [w448 w492] -> w347
                  frame No Error {
                    w447 = 2 ("length (rest)")
                    # "Initialize Lens Driver"
                    n234 = local read "Calibration"() -> (w439:T3)
                    n235 = for {
                      tunnel: w450 -> [w489]
                      tunnel: [w486] -> w442
                      tunnel: string[] ["Start", "MwDA", "CrMA00", "CrMB00", "CrUA00", "CrUB00", "CrLA00", "CrLB00", "PwTA\u0002Ð\u0001@"] -> [w484] mode=indexing
                      tunnel: [w483] -> w441
                      shift-right: [w487] -> w443
                      shift-left: w439 -> [w488]
                      shift-right: [w485] -> w444
                      shift-left: w451 -> [w490]
                      n236 = call "write read Lens Driver.vi"("VISA resource name"=w489, "command"=w484, "Calibration"=w488, "error in (no error)"=w490) -> ("VISA resource name out"=w486:refnum<visa-resource-name>, "Calibration 2"=w487:T3, "Data"=w483:string, "error out"=w485:errorcluster)  [unwired: 4 in, 4 out]
                    }
                    n237 = String Subset(string=w441, offset (0)=w447, length (rest)=w447) -> (substring=w445:string)
                    n238 = Type Cast(type=u16 0 ("length (rest)"), x=w445) -> (*(type *) &x=w440:u16)
                    n239 = local write "ID"(w440) -> ()
                    n240 = while {
                      tunnel: [w453] -> w449
                      tunnel: [w454] -> w448
                      tunnel: w444 -> [w459]
                      tunnel: w443 -> [w458]
                      tunnel: w442 -> [w457]
                      stop <- w452 stop-if-true
                      # "When Send command is true, Current Ch A is sent to the Lens Driver, in the correct format. If answer exists it is displayed in Data. The update rate of the while loop is 2ms."
                      n241 = Wait Until Next ms Multiple(millisecond multiple=u32 2) -> ()  [unwired: 1 out]
                      n242 = case shown="True" TRUE ("Send command") {
                        tunnel: [w461 w482] -> w453
                        tunnel: w459 -> [w461 w481]
                        tunnel: w458 -> [_ w469]
                        tunnel: w457 -> [w460 w480]
                        tunnel: [w460 w470] -> w454
                        frame False {
                        }
                        frame True {
                          n243 = Unbundle By Name(w469) -> ("Max Current A"=w468:dbl)
                          n244 = Multiply(x=15.8, y="Potencia inicial lente izquierdo") -> (x*y=w466:dbl)
                          n245 = Add(x=-6.8, y=w466) -> (x+y=w464:dbl)
                          n246 = Divide(x=w464, y=w468) -> (x/y=w467:dbl)
                          n247 = Multiply(x=4096.0, y=w467) -> (x*y=w478:dbl)
                          n248 = To Word Integer(number=w478) -> (16bit integer=w477:i16)
                          n249 = Type Cast(x=w477) -> (*(type *) &x=w476:string)  [unwired: 1 in]
                          n250 = Concatenate Strings("Aw", w476) -> (w472:string)
                          n251 = local write "Command to Port"(w472) -> ()
                          n252 = call "write read Lens Driver.vi"("VISA resource name"=w480, "command"=w472, "Calibration"=w469, "error in (no error)"=w481) -> ("VISA resource name out"=w470:refnum<visa-resource-name>, "Calibration 2"=w474:T3, "OK"=w473:bool, "Data"=w471:string, "error out"=w482:errorcluster)  [unwired: 4 in, 3 out]
                          n253 = local write "VISA resource name out 2"(w470) -> ()
                          n254 = local write "Calibration 2"(w474) -> ()
                          n255 = local write "Data"(w471) -> ()
                          n256 = local write "OK"(w473) -> ()
                          "DPT INICIALES I" <- "Potencia inicial lente izquierdo"
                        }
                      }
                      n257 = local read "Parar adquisicion"() -> (w452:bool)
                    }
                  }
                  frame Error {
                  }
                }
                n258 = VISA Close(VISA resource name=w347, error in (no error)=w348) -> (error out=w350:errorcluster)
                n259 = call <vilib>:"Simple Error Handler.vi"("error in (no error)"=w350) -> ("error out"=→"error out 4":errorcluster)  [unwired: 4 in, 4 out]
              }
              frame 1 {
                # "Mensaje que pregunta si desea realizar el experimento\ncon un nuevo usuario o con el actual"
                # "Se vuelven 0 los valores del WL y de la potencia óptica y distancia"
                # "En esta opcion se activa el modo experimento"
                n260 = property on="Waveform length" class="WFChart (strict)"("History Data"=dbl[][] [[0.0]]) -> ()  [unwired: 2 in, 2 out]
                n261 = property on="Potencia optica y distancia" class="WFChart (strict)"("History Data"=dbl[][] [[0.0]]) -> ()  [unwired: 2 in, 2 out]
                n262 = Two Button Dialog(message="Con quien desea realizar los experimentos?", 1:"Nuevo voluntario" ("F button name (\"Cancel\")"), 2:"Voluntario actual" ("T button name (\"OK\")")) -> (T button?=w511:bool)
                n263 = flat-sequence {
                  tunnel: w511 -> [w524]
                  tunnel: [w523] -> w509
                  tunnel: w508 -> [w523]
                  tunnel: [w516] -> w496
                  tunnel: w495 -> [w516]
                  tunnel: [w534] -> w512
                  tunnel: [w536] -> w510
                  tunnel: w509 -> [w536]
                  tunnel: [w535] -> w506
                  tunnel: w505 -> [w535]
                  tunnel: [w533] -> w497
                  tunnel: w496 -> [w533]
                  tunnel: w512 -> [w548]
                  tunnel: w510 -> [w547]
                  tunnel: [w546] -> w507
                  tunnel: w506 -> [w545]
                  tunnel: [w544] -> w503
                  tunnel: [w543] -> w502
                  tunnel: [w542] -> w500
                  tunnel: [w541] -> w498
                  tunnel: w497 -> [w541]
                  tunnel: w503 -> [w600]
                  tunnel: w502 -> [w583]
                  tunnel: [w600] -> w501
                  tunnel: w500 -> [w586]
                  tunnel: [w573] -> w499
                  tunnel: w498 -> [w573]
                  tunnel: [w603] -> w504
                  tunnel: w501 -> [w603]
                  tunnel: w499 -> [w601]
                  frame #0 {
                    # "Se guardan los datos de un nuevo voluntario"
                    n264 = Not(x=w524) -> (.not. x?=w518:bool)
                    n265 = case shown="False" w518 {
                      tunnel: [w527 w532] -> w522
                      tunnel: [w526 w531] -> w521
                      tunnel: [w528 w530] -> w520
                      tunnel: [w525 w529] -> w519
                      frame False {
                        n266 = local read "Enfermedad visual"() -> (w527:string)
                        n267 = local read "Nombre"() -> (w528:string)
                        n268 = local read "Cedula"() -> (w525:string)
                        n269 = local read "Edad"() -> (w526:string)
                      }
                      frame True {
                        n270 = call "Registro voluntario"() -> ("Enfermedad visual"=w532:string, "Edad"=w531:string, "Cedula"=w529:string, "Nombre"=w530:string)  [unwired: 14 in, 2 out]
                      }
                    }
                    "Cedula" <- w519
                    "Nombre" <- w520
                    "Edad" <- w521
                    "Enfermedad visual" <- w522
                    n271 = local write "T button?"(FALSE ("T button?")) -> ()
                  }
                  frame #1 {
                    n272 = Two Button Dialog(message="Qué tipo de experimento desea realizar?", 1:"Nuevo Experimento" ("F button name (\"Cancel\")"), 2:"Experimento existente" ("T button name (\"OK\")")) -> (T button?=w537:bool)
                    n273 = Not(x=w537) -> (.not. x?=w534:bool)
                  }
                  frame #2 {
                    # "A partir de la seleccion del experimento, se obtiene la descripcion correspondiente que será guardada en el archivo"
                    n274 = case shown="False" w548 {
                      tunnel: w547 -> [w550 w568]
                      tunnel: [w550 w567] -> w546
                      tunnel: w545 -> [w552 w566]
                      tunnel: [w552 w565] -> w544
                      tunnel: [w553 w564] -> w543
                      tunnel: [w549 w563] -> w542
                      frame False {
                        n275 = call "Display Message to User"() -> ()  [unwired: 10 in, 2 out]
                        n276 = flat-sequence {
                          tunnel: [w554] -> w551
                          tunnel: w550 -> [w554]
                          tunnel: [w562] -> w553
                          tunnel: w552 -> [w561]
                          tunnel: ["Menu experimentos"] -> _
                          tunnel: w551 -> [w559]
                          tunnel: [w558] -> w549
                          frame #0 {
                            n277 = while {
                              stop <- w555 stop-if-true
                              # "El sistema se queda en el loop hasta que el usuario elija el experimento que desea realizar"
                              n278 = event shown="[0] \"Elegir menu Exp\": Value Change" {
                                selector: _ -> [_ _]
                                dyn-events: _ -> [_ _]
                                timeout: _ -> [_ _]
                                tunnel: [TRUE FALSE] -> w555
                                event "Elegir menu Exp": Value Change {
                                n279 = event-data() -> ()  [unwired: 1 in, 4 out]
                                }
                                event Timeout {
                                n280 = event-data() -> ()  [unwired: 1 in, 3 out]
                                }
                              }
                            }
                          }
                          frame #1 {
                            n281 = Index Array(array=w561, index="Menu experimentos") -> (element=w562:string)
                            n282 = Index Array(array=w559, index="Menu experimentos") -> (element=w558:string)
                          }
                        }
                      }
                      frame True {
                        # "Se añade el nuevo experimento al menu de seleccion de experimentos"
                        # "Se guarda el nuevo experimento en el archivo que los contiene"
                        n283 = call "Nuevo experimento"() -> ("Descripcion"=w564:string, "Nombre"=w563:string)  [unwired: 16 in, 2 out]
                        n284 = Insert Into Array(array=w566, new element=w564) -> (w565:string[])  [unwired: 1 in]
                        n285 = Insert Into Array(array=w568, new element=w563) -> (w567:string[])  [unwired: 1 in]
                        n286 = property on="Menu experimentos" class="Ring (strict)"("Strings []"=w567) -> ()  [unwired: 2 in, 2 out]
                        n287 = Insert Into Array(array=string[] [], new element #1=w563, new element #2=w564) -> (w570:string[])  [unwired: 1 in]
                        n288 = call-poly <vilib>:"Write Delimited Spreadsheet.vi"("file path (dialog if empty)"=path "C:/Users/TGM1603/Documents/LabVIEW Data/Experimentos_realizados", "1D data"=w570, "append to file? (new file:F)"=TRUE) -> ()  [unwired: 11 in, 2 out]
                      }
                    }
                  }
                  frame #3 {
                    # "Se guardan los datos generales del experimento en el archivo de excel"
                    n289 = local read "Frecuencia muestreo"() -> (w575:i32)
                    n290 = local read "factor decimacion"() -> (w582:i32)
                    n291 = local read "Enfermedad visual"() -> (w585:string)
                    n292 = local read "Cedula"() -> (w587:string)
                    n293 = local read "Edad"() -> (w584:string)
                    n294 = local read "Rango voltaje"() -> (w579:i16)
                    n295 = local read "Nombre"() -> (w588:string)
                    n296 = Get Date/Time In Seconds() -> (seconds since 1Jan1904=w599:timestamp)
                    n297 = Path To String(path="Carpeta") -> (string=w595:string)
                    n298 = Format Date/Time String(time format string (%c)="_%d-%m-%y_%H-%M", seconds (now)=w599) -> (date/time string=w597:string)  [unwired: 1 in]
                    n299 = Number To Fractional String(number=w579, precision (6)=i16 0) -> (F-format string=w578:string)  [unwired: 2 in]
                    n300 = Number To Fractional String(number=w582, precision (6)=i16 0) -> (F-format string=w581:string)  [unwired: 2 in]
                    n301 = local read "Cedula"() -> (w591:string)
                    n302 = Number To Fractional String(number=w575, precision (6)=i16 0) -> (F-format string=w576:string)  [unwired: 2 in]
                    n303 = Concatenate Strings(w595, "\\" ("string"), w591, w597, "_" ("string"), w586, ".xlsx" ("string")) -> (w593:string)
                    n304 = String To Path(string=w593) -> (path=w592:path)
                    "path" <- w592
                    n305 = call "MS Office Report"("Path to Save Report"=w592, "Cedula"=w587, "decimacion"=w581, "Edad"=w584, "Enfermedad"=w585, "Exp_nombre"=w586, "Experimento"=w583, "freq"=w576, "Nombre"=w588, "rango"=w578) -> ()  [unwired: 16 in, 2 out]
                  }
                  frame #4 {
                    n306 = while {
                      shift-right: [w605] -> _
                      shift-left: enum16{"Inicio", "Tomar datos", ""}."Inicio" -> [w607]
                      tunnel: w601 -> [w604]
                      stop <- w606 stop-if-true
                      n307 = case shown="\"Tomar datos\"" w607 {
                        tunnel: [w608 w619] -> w605
                        tunnel: w604 -> [_ w614]
                        frame "Inicio", Default {
                          # "Se chequea si el usuario ha presionado el boton de comenzar el experimento. Si no lo ha hecho, se queda en este estado (0).\n Cuando lo presiona, pasa al estado de adquirir datios (1) ."
                          n308 = Select(t=enum16{"Inicio", "Tomar datos", ""}."Tomar datos", s="Iniciar experimento", f=enum16{"Inicio", "Tomar datos", ""}."Inicio") -> (s? t:f=w608:enum16{"Inicio", "Tomar datos", ""})
                        }
                        frame "Tomar datos" {
                          n309 = flat-sequence {
                            tunnel: [w703] -> w618
                            tunnel: [w702] -> w617
                            tunnel: [w701] -> w616
                            tunnel: [w700] -> w615
                            tunnel: w614 -> [w694]
                            tunnel: [w677] -> w613
                            tunnel: [w657] -> w612
                            tunnel: w618 -> [w1024]
                            tunnel: w617 -> [w1023]
                            tunnel: w616 -> [w1022]
                            tunnel: w615 -> [w1021]
                            tunnel: w613 -> [w1018]
                            tunnel: w612 -> [w1019]
                            tunnel: [enum16{"Inicio", "Tomar datos", ""}."Inicio"] -> w619
                            frame #0 {
                              w643 = u16 0 items=["None", "Last Bit", "TermChar", "Break"] ("Serial Settings:End Mode for Writes")
                              w644 = u16 2 items=["None", "Last Bit", "TermChar"] ("Serial Settings:End Mode for Reads")
                              w668 = u16 0 items=["None", "Last Bit", "TermChar", "Break"] ("Serial Settings:End Mode for Writes")
                              w669 = u16 2 items=["None", "Last Bit", "TermChar"] ("Serial Settings:End Mode for Reads")
                              w692 = 100  # max queue size
                              # "[9] Se unen en una sola matriz los vectores de tiempo, distancia, potencia derecha y potencia izquierda."
                              # "[9]"
                              # "[12] Se unen en una sola matriz, los vectores de  tiempo de la señal EMG, amplitud de la señal EMG, tiempo de potencia óptica, distancia, potencia óptica derecha y potencia óptica izquierda, en ese orden."
                              # "[8]"
                              # "[7]"
                              # "[6]"
                              # "[5]"
                              # "Se usan registros de desplazamiento para concatenar en un solo vector los datos que se obtienen en cada iteracion. Así en \n[1] Se guarda la potencia del lente derecho.\n[2] Por medio de variables locales, se guarda la distancia que se obtuvo en el bloque de distancia.\n[3]  Por medio de variables locales, se guarda la potencia del lente izquierdo que se obtuvo en el bloque de control de potencia del lente izquierdo.\n[4] Se guarda el tiempo actual.\n[5] Se pasa el vector de de potencia derecha a variable a string con 2 cifras significativas. \n[6] Se ajusta el vector del tiempo para que se muestre un tiempo relativo, es decir, en donde el primer dato sea 0 y en los demas se aumente un dt.  Además, se pasa el vector a variable a string con 5 cifras significativas.\n[7] Se pasa el vector de de distancia a variable a string con 0 cifras significativas. \n[8] Se pasa el vector de de potencia izquierda a variable a string con 2 cifras significativas."
                              # "En esta cola se guarda los datos de la señal EMG\nEn el bloque de adquisición los añade al adquirirlos y  en el de procesamiento los elimina al procesarlos ."
                              # "Initialize VISA port with correct parameters"
                              # "Initialize VISA port with correct parameters"
                              # "Close VISA port after program stop. Otherwise this port is blocked."
                              # "Se adquiere la señal del circuito de adquisicion, en donde se define la frecuencia de muestreo y el factor de decimacion.\n[1] Se inicializa el canal de adquisicion\n[2] Se ajusta el canal para que lea muestras continuas y apartir de estas prooduzca waveform data.\n[3]  Se obtiene los datos de la señal: la amplitud Y, el tiempo de inicio y el delta t.\n[4] Se decima el vector de amplitud. \n[5] Se usan registros de desplazamiento para concatenenar en un solo vector los datos de la amplitud que se obtienen en cada iteración. \n[6] Se obtiene el vector del tiempo."
                              # "[11] Los vectores de amplitud y tiempo se transforman a formato texto con 4 y 5 cifras significativas respectivamente y se unen para formar un vector de 2 columnas."
                              # "[9] Se ajusta el vector del tiempo para que se muestre un tiempo relativo, es decir, en donde el primer dato sea 0 y en los demas se aumente un dt. \n[10] Se extrae el primer elemento del vector ya que este siempre es 0 y no aporta información"
                              # "[12]"
                              # "[11]"
                              # "[10]"
                              # "[9]"
                              # "[8] Se guarda la fecha/hora en que se inicio el experimento"
                              # "[7] Se usan registros de desplazamiento para concatenar en un solo vector los datos del tiempo que se obtienen en cada iteracion."
                              # "Se define el rango de voltaje de adquisicon"
                              # "[1]"
                              n310 = while {
                                stop <- w738 stop-if-true
                                n311 = local read "Parar adquisicion"() -> (w733:bool)
                                n312 = call "grabarVideo.vi"("VideoMode"="Modo de video", "Quality"="Calidad", "Stop (F)"=w733, "Image Logging Path"="Carpeta archivo", "Frame Rate"="Frame Rate") -> ("Image Out"=→"Image Out":T1, "Stopped"=w738:bool)  [unwired: 20 in, 1 out]
                              }
                              n313 = local read "error in (no error)"() -> (w664:errorcluster)
                              n314 = local read "VISA resource name"() -> (w663:string)
                              n315 = local read "VISA resource name 2"() -> (w639:string)
                              n316 = call-poly "VISA Configure Serial Port"("VISA resource name"=w663, "timeout (10sec)"=u32 2000, "Enable Termination\nChar (T)"=FALSE ("Enable Termination\nChar (T)"), "baud rate (9600)"=u32 115200, "error in (no error)"=w664) -> ("VISA resource name out"=w673:refnum<visa-resource-name>, "error out"=w671:errorcluster)  [unwired: 9 in]
                              n317 = call-poly "VISA Configure Serial Port"("VISA resource name"=w639, "timeout (10sec)"=u32 2000, "Enable Termination\nChar (T)"=FALSE ("Enable Termination\nChar (T)"), "baud rate (9600)"=u32 115200, "error in (no error)"="error in (no error) 5") -> ("VISA resource name out"=w648:refnum<visa-resource-name>, "error out"=w646:errorcluster)  [unwired: 9 in]
                              n318 = property class="Instr"(reference=w673, error in=w671, "TermChar"=u8 10 ("Message Based Settings:Termination Character"), "ASRL End In"=w669, "ASRL End Out"=w668) -> (reference out=w672:refnum<visa-resource-name>, error out=w670:errorcluster)
                              n319 = property class="Instr"(reference=w648, error in=w646, "TermChar"=u8 10 ("Message Based Settings:Termination Character"), "ASRL End In"=w644, "ASRL End Out"=w643) -> (reference out=w647:refnum<visa-resource-name>, error out=w645:errorcluster)
                              n320 = VISA Set I/O Buffer Size(VISA resource name=w672, error in (no error)=w670) -> (VISA resource name out=w666:refnum<visa-resource-name>, error out=w665:errorcluster)  [unwired: 2 in]
                              n321 = VISA Set I/O Buffer Size(VISA resource name=w647, error in (no error)=w645) -> (VISA resource name out=w641:refnum<visa-resource-name>, error out=w640:errorcluster)  [unwired: 2 in]
                              n322 = local read "Rango voltaje"() -> (w715:i16)
                              n323 = VISA Flush I/O Buffer(VISA resource name=w666, error in (no error)=w665) -> (VISA resource name out=w662:refnum<visa-resource-name>, error out=w661:errorcluster)  [unwired: 1 in]
                              n324 = VISA Flush I/O Buffer(VISA resource name=w641, error in (no error)=w640) -> (VISA resource name out=w637:refnum<visa-resource-name>, error out=w636:errorcluster)  [unwired: 1 in]
                              n325 = local read "Frecuencia muestreo"() -> (w716:i32)
                              n326 = local read "DAQmx Physical Channel"() -> (w717:tag)
                              n327 = invoke on="Parar adquisicion" class="Bool (strict)" method="Reinit To Default"() -> ()  [unwired: 3 in, 3 out]
                              n328 = Obtain Queue(max queue size (-1, unlimited)=w692, element data type="Cola tipo 2") -> (queue out=w691:refnum<queue>)  [unwired: 3 in, 2 out]
                              n329 = Enqueue Element(queue=w694, element=0.0) -> (queue out=w697:refnum<queue>)  [unwired: 2 in, 2 out]
                              n330 = Multiply(x=-1.0 ("y"), y=w715) -> (x*y=w723:dbl)
                              n331 = call "Analog channel - inicializacion.vi"("maximum value"=w715, "minimum value"=w723, "rate"=w716, "DAQmx Physical Channel"=w717) -> ("error out"=w722:errorcluster, "task out"=w721:refnum<k21>)
                              n332 = local read "tamaño buffer"() -> (w718:i32)
                              n333 = call <vilib>:"DAQmx Start Task.vi"("task/channels in"=w721, "error in"=w722) -> ("task out"=w719:refnum<k21>, "error out"=w720:errorcluster)  [unwired: 12 in]
                              n334 = case shown="No Error" w636 {
                                tunnel: w636 -> [w754 w811]
                                tunnel: w637 -> [w753 w812]
                                tunnel: [w752 w811] -> w623
                                tunnel: [w751 w812] -> w622
                                tunnel: [w741 dbl[] [-30.0]] -> _
                                frame No Error {
                                w750 = 2 ("length (rest)")
                                # "Bloque de control del izquierdo. Se explica en el caso 0 de visualziación general"
                                # "Initialize Lens Driver"
                                n335 = local read "Calibration"() -> (w742:T3)
                                n336 = for {
                                tunnel: w753 -> [w808]
                                tunnel: [w805] -> w745
                                tunnel: string[] ["Start", "MwDA", "CrMA00", "CrMB00", "CrUA00", "CrUB00", "CrLA00", "CrLB00", "PwTA\u0002Ð\u0001@"] -> [w803] mode=indexing
                                tunnel: [w802] -> w744
                                shift-right: [w806] -> w746
                                shift-left: w742 -> [w807]
                                shift-right: [w804] -> w747
                                shift-left: w754 -> [w809]
                                n337 = call "write read Lens Driver.vi"("VISA resource name"=w808, "command"=w803, "Calibration"=w807, "error in (no error)"=w809) -> ("VISA resource name out"=w805:refnum<visa-resource-name>, "Calibration 2"=w806:T3, "Data"=w802:string, "error out"=w804:errorcluster)  [unwired: 4 in, 4 out]
                                }
                                n338 = String Subset(string=w744, offset (0)=w750, length (rest)=w750) -> (substring=w748:string)
                                n339 = Type Cast(type=u16 0 ("length (rest)"), x=w748) -> (*(type *) &x=w743:u16)
                                n340 = local write "ID"(w743) -> ()
                                n341 = while {
                                tunnel: [w759] -> w752
                                tunnel: [w760] -> w751
                                tunnel: w747 -> [w765]
                                tunnel: w746 -> [w764]
                                tunnel: w745 -> [w763]
                                shift-right: [w756] -> w741
                                shift-left: _ -> [w757]
                                stop <- w758 stop-if-true
                                # "When Send command is true, Current Ch A is sent to the Lens Driver, in the correct format. If answer exists it is displayed in Data. The update rate of the while loop is 2ms."
                                n342 = case shown="True" TRUE ("Send command") {
                                tunnel: [w771 w794] -> w759
                                tunnel: w765 -> [w771 w793]
                                tunnel: w764 -> [_ w774]
                                tunnel: w763 -> [w770 w792]
                                tunnel: [w770 w785] -> w760
                                tunnel: [dbl[] [-20.0] w784] -> w756
                                tunnel: w757 -> [_ w783]
                                frame False {
                                }
                                frame True {
                                n343 = local read "Potencia inicial lente izquierdo"() -> (w782:dbl)
                                n344 = local read "DPT dif."() -> (w781:dbl)
                                n345 = Add(x=w781, y=w782) -> (x+y=w777:dbl)
                                n346 = Absolute Value(x=w777) -> (abs(x)=w779:dbl)
                                n347 = Greater Or Equal?(x=6.0, y=w779) -> (x >= y?=w778:bool)
                                n348 = case shown="False" w778 {
                                tunnel: w777 -> [w797 w801]
                                tunnel: [w795 w801] -> w775
                                frame False {
                                n349 = Greater Or Equal?(x=u16 0, y=w797) -> (x >= y?=w798:bool)
                                n350 = case shown="False" w798 {
                                tunnel: [i16 6 ("x") i16 -6 ("x")] -> w795
                                frame False {
                                }
                                frame True {
                                }
                                }
                                }
                                frame True {
                                }
                                }
                                "Potencia izquierdo" <- w775
                                n351 = Unbundle By Name(w774) -> ("Max Current A"=w773:dbl)
                                n352 = call "potencia a corriente.vi"("Max current A"=w773, "Potencia"=w775) -> ("Corriente"=w776:dbl)
                                n353 = To Word Integer(number=w776) -> (16bit integer=w791:i16)
                                n354 = Type Cast(x=w791) -> (*(type *) &x=w790:string)  [unwired: 1 in]
                                n355 = Concatenate Strings("Aw", w790) -> (w787:string)
                                n356 = local write "Command to Port"(w787) -> ()
                                n357 = call "write read Lens Driver.vi"("VISA resource name"=w792, "command"=w787, "Calibration"=w774, "error in (no error)"=w793) -> ("VISA resource name out"=w785:refnum<visa-resource-name>, "Calibration 2"=w789:T3, "OK"=w788:bool, "Data"=w786:string, "error out"=w794:errorcluster)  [unwired: 4 in, 3 out]
                                n358 = local write "VISA resource name 2"(w785) -> ()
                                n359 = local write "Calibration 2"(w789) -> ()
                                n360 = local write "Data"(w786) -> ()
                                n361 = local write "OK"(w788) -> ()
                                n362 = Build Array (concatenate)(w783, w775) -> (w784:dbl[])
                                }
                                }
                                n363 = Wait Until Next ms Multiple(millisecond multiple=u32 10) -> ()  [unwired: 1 out]
                                n364 = local read "Parar adquisicion"() -> (w758:bool)
                                n365 = event shown="[0] \"Restablecer Iniciales\": Value Change" {
                                selector: _ -> [_ _]
                                dyn-events: _ -> [_ _]
                                timeout: 100 -> [_ _]
                                event "Restablecer Iniciales": Value Change {
                                n366 = event-data() -> ()  [unwired: 1 in, 3 out]
                                n367 = local read "Potencia inicial lente izquierdo"() -> (w766:dbl)
                                n368 = local read "Potencia inicial lente derecho"() -> (w767:dbl)
                                n369 = local write "Potencia izquierdo"(w766) -> ()
                                n370 = local write "Potencia derecho"(w767) -> ()
                                n371 = local write "DPT dif."(0.0 ("DPT dif.")) -> ()
                                }
                                event Timeout {
                                n372 = event-data() -> ()  [unwired: 1 in, 3 out]
                                }
                                }
                                }
                                }
                                frame Error {
                                }
                              }
                              n373 = case shown="No Error" w661 {
                                tunnel: w661 -> [w834 w930]
                                tunnel: w662 -> [w833 w931]
                                tunnel: [w832 w930] -> w689
                                tunnel: [w831 w931] -> w688
                                tunnel: [w820 dbl[] [-1.0]] -> w681
                                tunnel: [w819 dbl[] [-30.0]] -> w629
                                tunnel: [w818 u32[] [0]] -> w659
                                tunnel: [w816 dbl[] [-30.0]] -> w632
                                frame No Error {
                                w830 = 2 ("length (rest)")
                                # "Bloque de control del lente derecho. Se explica en el caso 0 de visualziación general"
                                # "Initialize Lens Driver"
                                n374 = local read "Calibration"() -> (w822:T3)
                                n375 = for {
                                tunnel: w833 -> [w924]
                                tunnel: [w921] -> w825
                                tunnel: string[] ["Start", "MwDA", "CrMA00", "CrMB00", "CrUA00", "CrUB00", "CrLA00", "CrLB00", "PwTA\u0002Ð\u0001@"] -> [w919] mode=indexing
                                tunnel: [w918] -> w824
                                shift-right: [w922] -> w826
                                shift-left: w822 -> [w923]
                                shift-right: [w920] -> w827
                                shift-left: w834 -> [w925]
                                n376 = call "write read Lens Driver.vi"("VISA resource name"=w924, "command"=w919, "Calibration"=w923, "error in (no error)"=w925) -> ("VISA resource name out"=w921:refnum<visa-resource-name>, "Calibration 2"=w922:T3, "Data"=w918:string, "error out"=w920:errorcluster)  [unwired: 4 in, 4 out]
                                }
                                n377 = String Subset(string=w824, offset (0)=w830, length (rest)=w830) -> (substring=w828:string)
                                n378 = Type Cast(type=u16 0 ("length (rest)"), x=w828) -> (*(type *) &x=w823:u16)
                                n379 = local write "ID"(w823) -> ()
                                n380 = while {
                                tunnel: [w852] -> w832
                                tunnel: [w853] -> w831
                                tunnel: w827 -> [w858]
                                tunnel: w826 -> [w857]
                                tunnel: w825 -> [w856]
                                shift-right: [w839] -> w820
                                shift-left: dbl[] [0.0] -> [w840]
                                shift-right: [w847] -> w819
                                shift-left: dbl[] [0.0] -> [w850]
                                shift-right: [w846] -> w818
                                shift-left: u32[] [0] -> [w849]
                                shift-right: [w837] -> w816
                                shift-left: dbl[] [0.0] -> [w836]
                                stop <- w851 stop-if-true
                                # "[4]"
                                # "[3]"
                                # "[2]"
                                # "When Send command is true, Current Ch A is sent to the Lens Driver, in the correct format. If answer exists it is displayed in Data. The update rate of the while loop is 2ms."
                                n381 = Wait Until Next ms Multiple(millisecond multiple=u32 10) -> ()  [unwired: 1 out]
                                n382 = case shown="True" TRUE ("Send command") {
                                tunnel: [w865 w884] -> w852
                                tunnel: w858 -> [w865 w883]
                                tunnel: w857 -> [_ w868]
                                tunnel: w856 -> [w864 w882]
                                tunnel: [w864 w874] -> w853
                                tunnel: [dbl[] [-20.0] w873] -> w847
                                tunnel: w850 -> [_ w872]
                                frame False {
                                }
                                frame True {
                                # "[1]"
                                n383 = local read "number"() -> (w879:u32)
                                n384 = local read "Potencia inicial lente derecho"() -> (w871:dbl)
                                n385 = case shown="2" w879 {
                                tunnel: [w885 w894 w909] -> w870
                                tunnel: w871 -> [w887 w889 w904]
                                tunnel: w871 -> [_ w888 w903]
                                frame 0, Default {
                                n386 = local read "DPT dif."() -> (w886:dbl)
                                n387 = Add(x=w887, y=w886) -> (x+y=w885:dbl)
                                }
                                frame 1 {
                                n388 = local read "DPT dif."() -> (w890:dbl)
                                n389 = Add(x=w889, y=w890) -> (x+y=w891:dbl)
                                n390 = Less Or Equal?(x=w891, y=6.0) -> (x <= y?=w893:bool)
                                n391 = case shown="True" w893 {
                                tunnel: [w896 w900] -> w894
                                tunnel: w888 -> [w895 w899]
                                frame False {
                                n392 = local read "DPT dif."() -> (w897:dbl)
                                n393 = Add(x=w895, y=w897) -> (x+y=w896:dbl)
                                }
                                frame True {
                                n394 = local read "DPT dif."() -> (w901:dbl)
                                n395 = local read "Incremento"() -> (w898:dbl)
                                n396 = Add(x=w901, y=w898) -> (x+y=w902:dbl)
                                n397 = local write "DPT dif."(w902) -> ()
                                n398 = Add(x=w899, y=w902) -> (x+y=w900:dbl)
                                }
                                }
                                }
                                frame 2 {
                                n399 = local read "DPT dif."() -> (w908:dbl)
                                n400 = Add(x=w908, y=w904) -> (x+y=w905:dbl)
                                n401 = Greater Or Equal?(x=w905, y=-6.0) -> (x >= y?=w906:bool)
                                n402 = case shown="True" w906 {
                                tunnel: [w911 w915] -> w909
                                tunnel: w903 -> [w910 w914]
                                frame False {
                                n403 = local read "DPT dif."() -> (w912:dbl)
                                n404 = Add(x=w910, y=w912) -> (x+y=w911:dbl)
                                }
                                frame True {
                                n405 = local read "DPT dif."() -> (w917:dbl)
                                n406 = local read "Incremento"() -> (w913:dbl)
                                n407 = Subtract(x=w917, y=w913) -> (x-y=w916:dbl)
                                n408 = local write "DPT dif."(w916) -> ()
                                n409 = Add(x=w914, y=w916) -> (x+y=w915:dbl)
                                }
                                }
                                }
                                }
                                "Potencia derecho" <- w870
                                n410 = Unbundle By Name(w868) -> ("Max Current A"=w867:dbl)
                                n411 = call "potencia a corriente.vi"("Max current A"=w867, "Potencia"=w870) -> ("Corriente"=w869:dbl)
                                n412 = To Word Integer(number=w869) -> (16bit integer=w881:i16)
                                n413 = Type Cast(x=w881) -> (*(type *) &x=w880:string)  [unwired: 1 in]
                                n414 = Concatenate Strings("Aw", w880) -> (w876:string)
                                n415 = local write "Command to Port"(w876) -> ()
                                n416 = call "write read Lens Driver.vi"("VISA resource name"=w882, "command"=w876, "Calibration"=w868, "error in (no error)"=w883) -> ("VISA resource name out"=w874:refnum<visa-resource-name>, "Calibration 2"=w878:T3, "OK"=w877:bool, "Data"=w875:string, "error out"=w884:errorcluster)  [unwired: 4 in, 3 out]
                                n417 = local write "VISA resource name out"(w874) -> ()
                                n418 = local write "Calibration 2"(w878) -> ()
                                n419 = local write "Data"(w875) -> ()
                                n420 = local write "OK"(w877) -> ()
                                n421 = Build Array (concatenate)(w872, w870) -> (w873:dbl[])
                                }
                                }
                                n422 = local read "Parar adquisicion"() -> (w851:bool)
                                n423 = local read "Potencia izquierdo"() -> (w835:dbl)
                                n424 = local read "Distancia"() -> (w848:u32)
                                n425 = property on="Potencia optica y distancia" class="WFChart (strict)"("YScale.ScaleFit"="Auto scale Y") -> ()  [unwired: 2 in, 2 out]
                                n426 = Get Date/Time In Seconds() -> (seconds since 1Jan1904=w841:timestamp)
                                n427 = To Double Precision Float(number=w841) -> (double precision float=w838:dbl)
                                n428 = property on="Potencia optica y distancia" class="WFChart (strict)"("XScale.ScaleFit"="Auto scale X") -> ()  [unwired: 2 in, 2 out]
                                n429 = Build Array (concatenate)(w840, w838) -> (w839:dbl[])
                                n430 = case shown="0, Default" "Auto scale Y" {
                                frame 0, Default {
                                n431 = property on="Potencia optica y distancia" class="WFChart (strict)"("YScale.Maximum"="Escala Y max") -> ()  [unwired: 2 in, 2 out]
                                n432 = property on="Potencia optica y distancia" class="WFChart (strict)"("YScale.Minimum"="Escala Y min") -> ()  [unwired: 2 in, 2 out]
                                }
                                frame 1 {
                                }
                                }
                                n433 = Build Array (concatenate)(w836, w835) -> (w837:dbl[])
                                n434 = Build Array (concatenate)(w849, w848) -> (w846:u32[])
                                n435 = case shown="0, Default" "Auto scale X" {
                                frame 0, Default {
                                n436 = property on="Potencia optica y distancia" class="WFChart (strict)"("XScale.Maximum"="Escala X max") -> ()  [unwired: 2 in, 2 out]
                                n437 = property on="Potencia optica y distancia" class="WFChart (strict)"("XScale.Minimum"="Escala X min") -> ()  [unwired: 2 in, 2 out]
                                }
                                frame 1 {
                                }
                                }
                                n438 = Build Array(w847, w846) -> (w845:dbl[][])
                                n439 = Transpose 2D Array(2D array=w845) -> (transposed array=→"Potencia optica y distancia":dbl[][])
                                }
                                }
                                frame Error {
                                }
                              }
                              n440 = while {
                                tunnel: w697 -> [w963]
                                shift-right: [w965] -> _
                                shift-left: dbl[] [0.0] -> [w971]
                                shift-right: [w964] -> _
                                shift-left: u32[] [0] -> [w966]
                                tunnel: [w963] -> w695
                                tunnel: w691 -> [w955]
                                stop <- w954 stop-if-true
                                # "Bloque de procesamiento.  Se explica en el caso 0 de visualización general"
                                n441 = local read "WL"() -> (w962:dbl)
                                n442 = local read "Parar adquisicion"() -> (w954:bool)
                                n443 = local read "Limite superior WL"() -> (w959:dbl)
                                n444 = call "waveform_length.vi"("WL"=w962, "Cola WL"=w963, "Datos entrada"=w955) -> ("WL 2"=w970:dbl)
                                n445 = local read "Limite inferior WL"() -> (w961:dbl)
                                n446 = local write "WL"(w970) -> ()
                                n447 = Build Array (concatenate)(w971, w970) -> (w965:dbl[])
                                n448 = In Range and Coerce(upper limit=w959, x=w970, lower limit=w961) -> (In Range?=w968:bool)  [unwired: 1 out]
                                n449 = Greater?(x=w970, y=w959) -> (0:w969:bool)
                                n450 = local read "Escala autom. X"() -> (w956:u8)
                                n451 = local read "Escala autom. Y"() -> (w957:u8)
                                n452 = Build Array(w969, w968) -> (w967:bool[])
                                n453 = Boolean Array To Number(Boolean array=w967) -> (number=w960:u32)
                                n454 = local write "number"(w960) -> ()
                                n455 = Build Array (concatenate)(w966, w960) -> (w964:u32[])
                                n456 = Build Array(w965, w964) -> (w958:dbl[][])
                                n457 = Transpose 2D Array(2D array=w958) -> (transposed array=w953:dbl[][])
                                n458 = local write "Waveform length"(w953) -> ()
                                n459 = property on="Waveform length" class="WFChart (strict)"("XScale.ScaleFit"=w956) -> ()  [unwired: 2 in, 2 out]
                                n460 = property on="Waveform length" class="WFChart (strict)"("YScale.ScaleFit"=w957) -> ()  [unwired: 2 in, 2 out]
                                n461 = case shown="0, Default" w957 {
                                frame 0, Default {
                                n462 = local read "Maximo escala Y"() -> (w975:dbl)
                                n463 = local read "Minimo escala Y"() -> (w974:dbl)
                                n464 = property on="Waveform length" class="WFChart (strict)"("YScale.Maximum"=w975) -> ()  [unwired: 2 in, 2 out]
                                n465 = property on="Waveform length" class="WFChart (strict)"("YScale.Minimum"=w974) -> ()  [unwired: 2 in, 2 out]
                                }
                                frame 1 {
                                }
                                }
                                n466 = case shown="0, Default" w956 {
                                frame 0, Default {
                                n467 = local read "Maximo escala X"() -> (w972:dbl)
                                n468 = local read "Minimo escala X"() -> (w973:dbl)
                                n469 = property on="Waveform length" class="WFChart (strict)"("XScale.Maximum"=w972) -> ()  [unwired: 2 in, 2 out]
                                n470 = property on="Waveform length" class="WFChart (strict)"("XScale.Minimum"=w973) -> ()  [unwired: 2 in, 2 out]
                                }
                                frame 1 {
                                }
                                }
                              }
                              n471 = while {
                                tunnel: w719 -> [w1008]
                                tunnel: w718 -> [w1005]
                                tunnel: [w1006] -> w705
                                shift-right: [w1003] -> w704
                                shift-left: w720 -> [w1007]
                                tunnel: [w998] -> w732
                                shift-right: [w997] -> w702
                                shift-left: _ -> [w996]
                                shift-right: [w987] -> w707
                                shift-left: dbl[] [0.0] -> [w992]
                                shift-right: [w988] -> w712
                                shift-left: dbl[] [0.0] -> [w989]
                                tunnel: w691 -> [w980]
                                i -> [w999]
                                stop <- w1002 stop-if-true
                                w1001 = 10.0  # timeout (s)
                                # "[7]"
                                # "[6]"
                                # "[5]"
                                # "[4]"
                                # "[3]"
                                # "[2]"
                                n472 = local read "Escala automatica X"() -> (w978:u8)
                                n473 = local read "Escala automatica Y"() -> (w977:u8)
                                n474 = property on="Senal EMG" class="WFGraph (strict)"("XScale.ScaleFit"=w978) -> ()  [unwired: 2 in, 2 out]
                                n475 = case shown="0, Default" w978 {
                                frame 0, Default {
                                n476 = local read "X Scale.Range:Increment"() -> (w1011:dbl)
                                n477 = local read "X Scale.Range:Maximum"() -> (w1013:dbl)
                                n478 = local read "X Scale.Range:Minimum"() -> (w1012:dbl)
                                n479 = property on="Senal EMG" class="WFGraph (strict)"("XScale.Increment"=w1011) -> ()  [unwired: 2 in, 2 out]
                                n480 = property on="Senal EMG" class="WFGraph (strict)"("XScale.Minimum"=w1012) -> ()  [unwired: 2 in, 2 out]
                                n481 = property on="Senal EMG" class="WFGraph (strict)"("XScale.Maximum"=w1013) -> ()  [unwired: 2 in, 2 out]
                                }
                                frame 1 {
                                }
                                }
                                n482 = local read "Parar adquisicion"() -> (w983:bool)
                                n483 = call-poly <vilib>:"DAQmx Read.vi"("task/channels in"=w1008, "number of samples per channel"=w1005, "timeout"=w1001, "error in"=w1007) -> ("task out"=w1006:refnum<k21>, "data"=w993:waveform(dbl)[], "error out"=w1003:errorcluster)  [unwired: 9 in]
                                n484 = Unbundle By Name(w1003) -> ("status"=w1004:bool)
                                n485 = Or(x=w1004, y=w983) -> (x .or. y?=w1002:bool)
                                n486 = property on="Senal EMG" class="WFGraph (strict)"("YScale.ScaleFit"=w977) -> ()  [unwired: 2 in, 2 out]
                                n487 = local write "Senal EMG"(w993) -> ()
                                n488 = case shown="0, Default" w977 {
                                frame 0, Default {
                                n489 = local read "Y Scale.Range:Maximum"() -> (w1010:dbl)
                                n490 = local read "Y Scale.Range:Minimum"() -> (w1009:dbl)
                                n491 = property on="Senal EMG" class="WFGraph (strict)"("YScale.Minimum"=w1009) -> ()  [unwired: 2 in, 2 out]
                                n492 = property on="Senal EMG" class="WFGraph (strict)"("YScale.Maximum"=w1010) -> ()  [unwired: 2 in, 2 out]
                                }
                                frame 1 {
                                }
                                }
                                n493 = call-poly <vilib>:"Index Waveform Array.vi"("index"=0, "waveform array"=w993) -> ("waveform"=w991:waveform(dbl))  [unwired: 8 in, 1 out]
                                n494 = Unbundle By Name(w991) -> ("Y"=w981:dbl[], "t0"=w998:timestamp)  [unwired: 1 out]
                                n495 = call-poly <vilib>:"Decimate (continuous).vi"("averaging"=TRUE, "decimating factor"="factor decimacion", "X"=w981) -> ("Decimated Array"=w976:dbl[])  [unwired: 7 in, 1 out]
                                n496 = Lossy Enqueue Element(queue=w980, element=w976) -> ()  [unwired: 1 in, 4 out]
                                n497 = Build Array (concatenate)(w992, w976) -> (w987:dbl[])
                                n498 = case shown="1" w999 {
                                tunnel: w998 -> [_ w1017]
                                tunnel: [w1015 w1016] -> w997
                                tunnel: w996 -> [w1015 _]
                                frame 0, Default {
                                }
                                frame 1 {
                                # "[8]"
                                n499 = Format Date/Time String(seconds (now)=w1017) -> (date/time string=w1016:string)  [unwired: 2 in]
                                }
                                }
                                n500 = local read "factor decimacion"() -> (w984:i32)
                                n501 = call-poly <vilib>:"Get Waveform Time Array.vi"("waveform in"=w991) -> ("X array"=w990:timestamp[])  [unwired: 9 in, 1 out]
                                n502 = event shown="[0] \"Ganancia\": Value Change" {
                                selector: _ -> [_ _]
                                dyn-events: _ -> [_ _]
                                timeout: 1 -> [_ _]
                                tunnel: "Ganancia" -> [w1014 _]
                                event "Ganancia": Value Change {
                                n503 = event-data() -> ()  [unwired: 1 in, 4 out]
                                n504 = call "Ganancia programable.vi"("MOSI data"=w1014) -> ()
                                }
                                event Timeout {
                                n505 = event-data() -> ()  [unwired: 1 in, 3 out]
                                }
                                }
                                n506 = To Double Precision Float(number=w990) -> (double precision float=w986:dbl[])
                                n507 = call-poly <vilib>:"Decimate (single shot).vi"("decimating factor"=w984, "X"=w986) -> ("Decimated Array"=w985:dbl[])  [unwired: 8 in, 1 out]
                                n508 = Build Array (concatenate)(w989, w985) -> (w988:dbl[])
                              }
                              n509 = call <vilib>:"DAQmx Clear Task.vi"("task in"=w705, "error in"=w704) -> ()  [unwired: 13 in, 1 out]
                              n510 = Index Array(array=w712, index=1) -> (element=w711:dbl)
                              n511 = Flush Queue(queue=w695) -> ()  [unwired: 1 in, 3 out]
                              n512 = Subtract(x=w712, y=w711) -> (x-y=w709:dbl[])
                              n513 = Delete From Array(array=w707, index=0) -> (array with subset deleted=w727:dbl[])  [unwired: 1 in, 1 out]
                              n514 = while {
                                shift-right: [w932] -> _
                                shift-left: _ -> [w933]
                                stop <- w937 stop-if-true
                                # "Este bloque adquiere la distancia (se explica en el caso 0 (visualizacion general)"
                                n515 = call "meididor de distancia archivo adicional.vi"() -> ("error out"=w940:errorcluster, "task out"=w941:refnum<k21>)  [unwired: 10 in]
                                n516 = call "DAQ Assistant2"("timeout (s)"=0.05) -> ("data"=w950:dynamicdata, "error out"=w938:errorcluster)  [unwired: 16 in, 1 out]
                                n517 = call <vilib>:"DAQmx Start Task.vi"("task/channels in"=w941, "error in"=w940) -> ("task out"=w944:refnum<k21>, "error out"=w945:errorcluster)  [unwired: 12 in]
                                n518 = call <vilib>:"DAQmx Is Task Done.vi"("task/channels in"=w944, "error in"=w945) -> ("task out"=w942:refnum<k21>, "error out"=w943:errorcluster)  [unwired: 11 in, 1 out]
                                n519 = Wait (ms)(milliseconds to wait=u32 200) -> ()  [unwired: 1 out]
                                n520 = call <vilib>:"Clear Errors.vi"("error in (no error)"=w938) -> ()  [unwired: 5 in, 2 out]
                                n521 = local read "Parar adquisicion"() -> (w937:bool)
                                n522 = call <vilib>:"DAQmx Clear Task.vi"("task in"=w942, "error in"=w943) -> ()  [unwired: 13 in, 1 out]
                                n523 = Multiply(x=1000000.0, y=w950) -> (x*y=w948:dynamicdata)
                                n524 = Divide(x=w948, y=58.0) -> (x/y=w934:dynamicdata)
                                n525 = Equal?(x=w934, y=0.0) -> (x = y?=w936:dynamicdata)
                                n526 = case shown="True" w936 {
                                tunnel: [w951 w952] -> w932
                                tunnel: w934 -> [w951 _]
                                tunnel: w933 -> [_ w952]
                                frame False {
                                }
                                frame True {
                                }
                                }
                                n527 = local write "Distancia"(w932) -> ()
                              }
                              n528 = Delete From Array(array=w709, index=0) -> (array with subset deleted=w726:dbl[])  [unwired: 1 in, 1 out]
                              n529 = local read "path"() -> (w703:path)
                              n530 = Format Date/Time String(seconds (now)=w732) -> (date/time string=w701:string)  [unwired: 2 in]
                              n531 = Number To Fractional String(use system decimal point (T)=FALSE, number=w727, precision (6)=i16 4) -> (F-format string=w655:string[])  [unwired: 1 in]
                              n532 = Number To Fractional String(use system decimal point (T)=FALSE, number=w726, precision (6)=i16 5) -> (F-format string=w656:string[])  [unwired: 1 in]
                              n533 = Build Array(w656, w655) -> (w725:string[][])
                              n534 = Transpose 2D Array(2D array=w725) -> (transposed array=w700:string[][])
                              n535 = Delete From Array(array=w629, index=0) -> (array with subset deleted=w628:dbl[])  [unwired: 1 in, 1 out]
                              n536 = Delete From Array(array=w659, index=0) -> (array with subset deleted=w625:u32[])  [unwired: 1 in, 1 out]
                              n537 = Index Array(array=w681, index=1) -> (element=w686:dbl)
                              n538 = Delete From Array(array=w632, index=0) -> (array with subset deleted=w631:dbl[])  [unwired: 1 in, 1 out]
                              n539 = VISA Close(VISA resource name=w622, error in (no error)=w623) -> (error out=w621:errorcluster)
                              n540 = Subtract(x=w681, y=w686) -> (x-y=w680:dbl[])
                              n541 = Number To Fractional String(use system decimal point (T)=FALSE, number=w628, precision (6)=i16 2) -> (F-format string=w652:string[])  [unwired: 1 in]
                              n542 = VISA Close(VISA resource name=w688, error in (no error)=w689) -> (error out=w690:errorcluster)
                              n543 = call <vilib>:"Simple Error Handler.vi"("error in (no error)"=w621) -> ("error out"=w620:errorcluster)  [unwired: 4 in, 4 out]
                              n544 = Number To Fractional String(number=w625, precision (6)=i16 0) -> (F-format string=w653:string[])  [unwired: 2 in]
                              n545 = Delete From Array(array=w680, index=0) -> (array with subset deleted=w685:dbl[])  [unwired: 1 in, 1 out]
                              n546 = call <vilib>:"Simple Error Handler.vi"("error in (no error)"=w690) -> ("error out"=w687:errorcluster)  [unwired: 4 in, 4 out]
                              n547 = Number To Fractional String(use system decimal point (T)=FALSE, number=w631, precision (6)=i16 2) -> (F-format string=w633:string[])  [unwired: 1 in]
                              n548 = local write "error out"(w687) -> ()
                              n549 = local write "error out"(w620) -> ()
                              n550 = Number To Fractional String(use system decimal point (T)=FALSE, number=w685, precision (6)=i16 5) -> (F-format string=w654:string[])  [unwired: 1 in]
                              n551 = Build Array(w656, w655, w654, w653, w652, w633) -> (w626:string[][])
                              n552 = Transpose 2D Array(2D array=w626) -> (transposed array=w657:string[][])
                              n553 = Build Array(w654, w653, w652, w633) -> (w677:string[][])
                            }
                            frame #1 {
                              # "[13]"
                              # "[13] En esta case structure, se decide que datos se van a guardar. Esto lo hace el SUBVI llamado guardar datos de amplitud y tiempo."
                              n554 = Transpose 2D Array(2D array=w1018) -> (transposed array=w1020:string[][])
                              n555 = call <vilib>:"Three Button Dialog.vi"("Right Button Text (\"Cancel\")"="Señal EMG, potencia optica y distancia" ("Right Button Text (\"Cancel\")"), "Center Button Text (\"No\")"="Potencia optica y distancia" ("Center Button Text (\"No\")"), "Left Button Text (\"Yes\")"="Señal EMG" ("Left Button Text (\"Yes\")"), "message"="Elija que datos desea guardar") -> ("Which Button?"=w1025:T4)  [unwired: 7 in]
                              n556 = case shown="\"Right Button\"" w1025 {
                                tunnel: w1024 -> [w1034 w1039 w1042]
                                tunnel: w1023 -> [w1033 w1038 w1043]
                                tunnel: w1022 -> [w1032 w1037 w1044]
                                tunnel: w1021 -> [w1031 _ _]
                                tunnel: w1020 -> [_ w1036 _]
                                tunnel: w1019 -> [_ _ w1040]
                                frame "Left Button", Default {
                                # "Se guarda solo la señal EMG y su tiempo de adquisición."
                                n557 = call "Guardar datos de Amplitud y Tiempo.vi"("path"=w1034, "Hora inicio"=w1033, "Hora fin"=w1032, "Datos experimento"=w1031, "column headers"=string[] ["Tiempo(s)", "Amplitud(V)"]) -> ()  [unwired: 1 in]
                                }
                                frame "Center Button" {
                                # "Se guarda la potenica del lente derecho, del lente izquierdo, la distancia y el tiempo de estas variables."
                                n558 = call "Guardar datos de Amplitud y Tiempo.vi"("path"=w1039, "Hora inicio"=w1038, "Hora fin"=w1037, "Datos experimento"=w1036, "column headers"=string[] ["Tiempo(s)", "Distancia (cm)", "Potencia Optica derecho", "Potencia optica izquierdo"]) -> ()  [unwired: 1 in]
                                }
                                frame "Right Button" {
                                # "Se guarda el tiempo de adquisición así como la amplitud de la señal EMG,  la potenica del lente derecho, del lente izquierdo, la distancia y el tiempo de estas variables."
                                n559 = call "Guardar datos de Amplitud y Tiempo.vi"("path"=w1042, "Hora inicio"=w1043, "Hora fin"=w1044, "Datos experimento"=w1040, "column headers"=string[] ["Tiempo EMG(s)", "Amplitud(V)", "Tiempo DPT(s)", "Distancia (cm)", "Potencia optica derecho", "Potencia optica izquierdo"]) -> ()  [unwired: 1 in]
                                }
                              }
                            }
                            frame #2 {
                              # "Si el usuario desea repetir el experimento se vuelve al estado inicio en donde se espera que comience el experimento. De lo contrario se sale del loop y vuelve al menu principal."
                              n560 = Two Button Dialog(message="¿Desea repetir el experimento?", 1:"No" ("F button name (\"Cancel\")"), 2:"Si" ("T button name (\"OK\")")) -> (T button?=w1047:bool)
                              n561 = Not(x=w1047) -> (.not. x?=→"T button?":bool)
                            }
                          }
                        }
                      }
                      n562 = local read "T button?"() -> (w606:bool)
                    }
                  }
                }
              }
            }
          }
          event Timeout {
            n563 = event-data() -> ()  [unwired: 1 in, 3 out]
          }
        }
      }
    }
  }
